vi "ACT_Loop.vi"() -> ()   [LabVIEW 2023, in "Swerve AM_ACT.lvlib"]
uses:
  Swerve AM_ACT.lvlib
  Cluster_CMD_ACT_Data.ctl
  ENUM_CMD_Mode Select.ctl
  Shared Code/TypeDefs/Cluster_CMD_Direction Data.ctl
  Shared Code/TypeDefs/Cluster_Module Velocity-Direction-Rotations.ctl
  Shared Code/TypeDefs/Level_Velocity plus-minus 1.ctl
  Shared Code/TypeDefs/Dial_Compase heading unit circle CCW positive.ctl
  Shared Code/TypeDefs/Cluster_X-Y.ctl
  Cluster_HW Output Values.ctl
  Shared Code/TypeDefs/Cluster_Swerve 4 Steer and Velocity.ctl
  Cluster_System Output Data.ctl
  Cluster_Config System Values.ctl
  Shared Code/TypeDefs/Cluster_SW PID Config.ctl
  Shared Code/TypeDefs/Cluster_PID Gains.ctl
  Shared Code/TypeDefs/Cluster_High-Low.ctl
  Type Defs/Cluster_Length and Width.ctl
  Shared Code/TypeDefs/Cluster_Config_SwerveParam Drive.ctl
  Shared Code/TypeDefs/Cluster_Config_SwerveParam Steer.ctl
  Cluster_Config Specific HW Values.ctl
  Cluster_Config Specific Data.ctl
  Shared Code/TypeDefs/ENUM_Module Position.ctl
  Cluster_Config Steer HW Values.ctl
  Shared Code/TypeDefs/Cluster_Config SRX Motor Output.ctl
  <vilib>/Rock Robotics/WPI/ThirdParty/Phoenix-LabVIEW/Motor Controller/Controls/CTRE_Phoenix_MotorControl_NeutralMode.ctl
  Shared Code/TypeDefs/Cluster_FWD  REV Values.ctl
  Shared Code/TypeDefs/Cluster_SRX SLOT PID Config.ctl
  Shared Code/TypeDefs/Cluster_SRX Motion Magic Parameters.ctl
  Cluster_Config Drive HW Values.ctl
  Shared Code/TypeDefs/Cluster_Spark MAX SLOT PID Config.ctl
  Shared Code/TypeDefs/Cluster_SparkMax Smart Motion Parameters.ctl
  ENUM_ACT_State.ctl
  <vilib>/Rock Robotics/WPI/ThirdParty/Phoenix-LabVIEW/Motor Controller/Controls/CTRE_Phoenix_MotorControl_ControlMode.ctl
  <vilib>/Rock Robotics/WPI/MotorControl/WPI_MotorControlDeviceRef.ctl
  <vilib>/Rock Robotics/WPI/MotorControl/WPI_MotorControlType.ctl
  <vilib>/Rock Robotics/SystemInterfaces/DIO/FPGA_DIOPWMChannel.ctl
  <vilib>/Rock Robotics/WPI/PWM/WPI_PWMDeadband.ctl
  <vilib>/Rock Robotics/SystemInterfaces/DIO/FPGA_DIOChannel.ctl
  ENUM_ACT_Action.ctl
  4f1f8321-3dc8-4b28-8619-20673fc77ec2.vi
  cbff3d61-3b62-444e-9844-795ae03579cd.vi
  089052c0-d540-4a78-a5cc-aeb70dbb496b.vi
  6201c2b1-dcd8-4430-86f1-9b4ee56c7753.vi
  b5508d6c-c1cc-4273-80c5-2077d34e1483.vi
  5f725c2a-0ce1-4524-8967-e83b15fdce90.vi
  bd5da564-2e8e-4505-86fc-30918feadaa2.vi
  8beda75f-c59a-4462-acc7-7c37ceab3777.vi
  47a9b741-f4a3-48b6-ae85-4ba2e502368e.vi
  e2e8a241-7810-4d95-85fd-17f3a55957a8.vi
  80d407e5-f582-430c-986f-ecd413765478.vi
  573e44c0-11f4-4bd9-ad56-904ec25dba75.vi
  e7494af9-f670-4352-9dfa-ae6ce50709ea.vi
  <vilib>/Utility/error.llb/Trim Whitespace.vi
  5f725c2a-0ce1-4524-8967-e83b15fdce90.vi/958b2683-dd4b-41b7-8ed1-41c95f63cef0.vi
  5f725c2a-0ce1-4524-8967-e83b15fdce90.vi/95f5fa9b-6175-4b34-88ee-cece92c38279.vi
  bd5da564-2e8e-4505-86fc-30918feadaa2.vi/958b2683-dd4b-41b7-8ed1-41c95f63cef0.vi
  bd5da564-2e8e-4505-86fc-30918feadaa2.vi/95f5fa9b-6175-4b34-88ee-cece92c38279.vi
  8beda75f-c59a-4462-acc7-7c37ceab3777.vi/958b2683-dd4b-41b7-8ed1-41c95f63cef0.vi
  8beda75f-c59a-4462-acc7-7c37ceab3777.vi/95f5fa9b-6175-4b34-88ee-cece92c38279.vi
  47a9b741-f4a3-48b6-ae85-4ba2e502368e.vi/958b2683-dd4b-41b7-8ed1-41c95f63cef0.vi
  47a9b741-f4a3-48b6-ae85-4ba2e502368e.vi/95f5fa9b-6175-4b34-88ee-cece92c38279.vi
  e2e8a241-7810-4d95-85fd-17f3a55957a8.vi/958b2683-dd4b-41b7-8ed1-41c95f63cef0.vi
  e2e8a241-7810-4d95-85fd-17f3a55957a8.vi/95f5fa9b-6175-4b34-88ee-cece92c38279.vi
  80d407e5-f582-430c-986f-ecd413765478.vi/958b2683-dd4b-41b7-8ed1-41c95f63cef0.vi
  80d407e5-f582-430c-986f-ecd413765478.vi/95f5fa9b-6175-4b34-88ee-cece92c38279.vi
  573e44c0-11f4-4bd9-ad56-904ec25dba75.vi/958b2683-dd4b-41b7-8ed1-41c95f63cef0.vi
  573e44c0-11f4-4bd9-ad56-904ec25dba75.vi/95f5fa9b-6175-4b34-88ee-cece92c38279.vi
  e7494af9-f670-4352-9dfa-ae6ce50709ea.vi/958b2683-dd4b-41b7-8ed1-41c95f63cef0.vi
  e7494af9-f670-4352-9dfa-ae6ce50709ea.vi/95f5fa9b-6175-4b34-88ee-cece92c38279.vi
  <vilib>/Utility/error.llb/Trim Whitespace One-Sided.vi
  5f725c2a-0ce1-4524-8967-e83b15fdce90.vi/95f5fa9b-6175-4b34-88ee-cece92c38279.vi/1c6bd52c-bbca-4d4a-a290-93ea2703fded.vi
  5f725c2a-0ce1-4524-8967-e83b15fdce90.vi/95f5fa9b-6175-4b34-88ee-cece92c38279.vi/47c2b0d5-b5fa-444e-9535-611565d375db.vi
  bd5da564-2e8e-4505-86fc-30918feadaa2.vi/95f5fa9b-6175-4b34-88ee-cece92c38279.vi/1c6bd52c-bbca-4d4a-a290-93ea2703fded.vi
  bd5da564-2e8e-4505-86fc-30918feadaa2.vi/95f5fa9b-6175-4b34-88ee-cece92c38279.vi/47c2b0d5-b5fa-444e-9535-611565d375db.vi
  8beda75f-c59a-4462-acc7-7c37ceab3777.vi/95f5fa9b-6175-4b34-88ee-cece92c38279.vi/1c6bd52c-bbca-4d4a-a290-93ea2703fded.vi
  8beda75f-c59a-4462-acc7-7c37ceab3777.vi/95f5fa9b-6175-4b34-88ee-cece92c38279.vi/47c2b0d5-b5fa-444e-9535-611565d375db.vi
  47a9b741-f4a3-48b6-ae85-4ba2e502368e.vi/95f5fa9b-6175-4b34-88ee-cece92c38279.vi/1c6bd52c-bbca-4d4a-a290-93ea2703fded.vi
  47a9b741-f4a3-48b6-ae85-4ba2e502368e.vi/95f5fa9b-6175-4b34-88ee-cece92c38279.vi/47c2b0d5-b5fa-444e-9535-611565d375db.vi
  e2e8a241-7810-4d95-85fd-17f3a55957a8.vi/95f5fa9b-6175-4b34-88ee-cece92c38279.vi/1c6bd52c-bbca-4d4a-a290-93ea2703fded.vi
  e2e8a241-7810-4d95-85fd-17f3a55957a8.vi/95f5fa9b-6175-4b34-88ee-cece92c38279.vi/47c2b0d5-b5fa-444e-9535-611565d375db.vi
  80d407e5-f582-430c-986f-ecd413765478.vi/95f5fa9b-6175-4b34-88ee-cece92c38279.vi/1c6bd52c-bbca-4d4a-a290-93ea2703fded.vi
  80d407e5-f582-430c-986f-ecd413765478.vi/95f5fa9b-6175-4b34-88ee-cece92c38279.vi/47c2b0d5-b5fa-444e-9535-611565d375db.vi
  573e44c0-11f4-4bd9-ad56-904ec25dba75.vi/95f5fa9b-6175-4b34-88ee-cece92c38279.vi/1c6bd52c-bbca-4d4a-a290-93ea2703fded.vi
  573e44c0-11f4-4bd9-ad56-904ec25dba75.vi/95f5fa9b-6175-4b34-88ee-cece92c38279.vi/47c2b0d5-b5fa-444e-9535-611565d375db.vi
  e7494af9-f670-4352-9dfa-ae6ce50709ea.vi/95f5fa9b-6175-4b34-88ee-cece92c38279.vi/1c6bd52c-bbca-4d4a-a290-93ea2703fded.vi
  e7494af9-f670-4352-9dfa-ae6ce50709ea.vi/95f5fa9b-6175-4b34-88ee-cece92c38279.vi/47c2b0d5-b5fa-444e-9535-611565d375db.vi
  RoboRIO Utilities/Global_STOP.vi
  Global_CMD_ACT_Data In.vi
  PigeonIMU/Global_SEN_Data Out.vi
  Global_ACT_Data Out.vi
  <vilib>/Utility/Data Type/Get Type Information.vi
  Shared Code/Utility/RWA/RWA/File/RWA_PC FIle Read String.vi
  Shared Code/Utility/RWA/RWA/Read Write Anything/RWA_File String.vi
  Shared Code/Utility/RWA/RWA/File/RWA_PC File Write String.vi
  <vilib>/Comparison/Equal/Equal Functor/Equal Functor.lvclass
  PigeonIMU/PigeonIMU_SEN_ts.lvlib
panel:
  in  "Set Steer Start Values":bool
  in  "Config Drive":T1={"Drive HW Ver"=0, "SparkMax Output"={"Idle Mode"=enum."Coast", "Ramp Rate (S)"=1.0}, "Slot 0 CL"={"Gains"={"P"=0.1, "I"=0.0, "D"=0.0, "F"=0.0}, "I Zone"=0.0, "Peak Out -1 0 1"={"High"=0.0, "Low"=0.0}, "Max I Accu"=0.0}, "Slot 0 SM"={"Max Velocity"=0.0, "Max Acceleration"=0.0, "Allowed CL Error"=0.0, "Min Velocity Output"=0.0}} {"Slot 0 CL"."Gains"."F" format="%#.8f"; "Slot 0 CL"."Gains"."D" format="%#.8f"; "Slot 0 CL"."Gains"."I" format="%#.8f"; "Slot 0 CL"."Gains"."P" format="%#.8f"; "Slot 0 CL"."Peak Out -1 0 1"."Low" format="%#.8f"; "Slot 0 CL"."Peak Out -1 0 1"."High" format="%#.8f"}
  in  "Config Steer":T6={"Steer HW Ver"=0, "SRX Output"={"Neutral"=enum."Override to Coast", "Max"={"FWD"=1.0, "REV"=-1.0}, "Min"={"FWD"=0.0, "REV"=0.0}, "OL Ramp Rate (S)"=0.0, "Dead Band"=0.0, "CL Ramp Rate (S)"=0.0}, "Slot 0 CL"={"Gains"={"P"=1.0, "I"=0.01, "D"=0.0, "F"=0.0}, "Error Allowed"=0.0, "I Zone"=10000.0, "Peak Out 0-1"=1.0, "Max I Accu"=-1000.0}, "Slot 0 MM"={"Cruise Velocity"=5000, "Acceleration"=5000}} {"Slot 0 CL"."Gains"."F" format="%#.8f"; "Slot 0 CL"."Gains"."D" format="%#.8f"; "Slot 0 CL"."Gains"."I" format="%#.8f"; "Slot 0 CL"."Gains"."P" format="%#.8f"; "SRX Output"."Min"."REV" format="%.2f"; "SRX Output"."Min"."FWD" format="%.2f"; "SRX Output"."Max"."REV" format="%.2f"; "SRX Output"."Max"."FWD" format="%.2f"}
  in  "Config Specific":T12={"Specific HW Ver"=0, "Specific Data"=[{"Motor Pos"=enum."Left-Front", "CAN Bus"="", "Drive ID"=0, "Drive Invert"=FALSE, "Steer ID"=0, "Steer Invert"=FALSE, "Encoder Start Value"=0.0}, {"Motor Pos"=enum."Right-Front", "CAN Bus"="", "Drive ID"=0, "Drive Invert"=FALSE, "Steer ID"=0, "Steer Invert"=FALSE, "Encoder Start Value"=0.0}, {"Motor Pos"=enum."Right-Back", "CAN Bus"="", "Drive ID"=0, "Drive Invert"=FALSE, "Steer ID"=0, "Steer Invert"=FALSE, "Encoder Start Value"=0.0}, {"Motor Pos"=enum."Left-Back", "CAN Bus"="", "Drive ID"=0, "Drive Invert"=FALSE, "Steer ID"=0, "Steer Invert"=FALSE, "Encoder Start Value"=0.0}]}
  in  "CMD Override":enum32{"None", "Mode 2", "Mode 1", "STOP"}(tab)
  in  "Mode 2 Data":dbl(slide) scale=-0.2..0.2
  in  "Mode 1 Data":i32
  in  "GO":bool
  out "Current Time":timestamp
  in  "Config System":T15={"System Ver"=0, "Auto Angle PID"={"Gains"={"P"=0.1, "I"=0.0, "D"=0.0, "F"=0.0}, "Error Allowed"={"High"=0.0, "Low"=0.0}, "I Zone"={"High"=0.0, "Low"=0.0}, "Peak Out 0-1"={"High"=0.0, "Low"=0.0}, "Max I Accu"={"High"=0.0, "Low"=0.0}}, "Frame"={"Length"=33.0, "Width"=18.0}, "DriveTrain"={"CPR"=14.0, "RevMotor/Wheel"=6.67, "Wheel Diameter (in)"=4.0}, "Speed Full Scale"=5000.0, "Steer Data"={"CPR"=1024.0}} {"Auto Angle PID"."Max I Accu"."Low" format="%#.8f"; "Auto Angle PID"."Max I Accu"."High" format="%#.8f"; "Auto Angle PID"."Gains"."F" format="%#.8f"; "Auto Angle PID"."Gains"."D" format="%#.8f"; "Auto Angle PID"."Gains"."I" format="%#.8f"; "Auto Angle PID"."Gains"."P" format="%#.8f"; "Auto Angle PID"."Error Allowed"."Low" format="%#.8f"; "Auto Angle PID"."Error Allowed"."High" format="%#.8f"; "Auto Angle PID"."I Zone"."Low" format="%#.8f"; "Auto Angle PID"."I Zone"."High" format="%#.8f"; "Auto Angle PID"."Peak Out 0-1"."Low" format="%#.8f"; "Auto Angle PID"."Peak Out 0-1"."High" format="%#.8f"}
  out "System Config":T20
  out "Sensor Read time":dbl format="%.3g"
  out "HW Output":T21 {"Swerve Read"."Back Right"."Angle" scale format="%.3f"; "Swerve Read"."Back Right"."Velocity" scale=-1.0..1.0 scale format="%.1f"; "Swerve Read"."Back Left"."Angle" scale format="%.3f"; "Swerve Read"."Back Left"."Velocity" scale=-1.0..1.0 scale format="%.1f"; "Swerve Read"."Front Left"."Angle" scale format="%.3f"; "Swerve Read"."Front Left"."Velocity" scale=-1.0..1.0 scale format="%.1f"; "Swerve Read"."Front Right"."Angle" scale format="%.3f"; "Swerve Read"."Front Right"."Velocity" scale=-1.0..1.0 scale format="%.1f"; "Pigeon Heading" scale format="%.3f"}
  in  "Read Saved Config":bool
  in  "Update Config":bool
  out "CMD":T26 {"Target Auto Angle" scale format="%.3f"; "Direction"."Rotate(Yaw) CCW 1 CW -1" scale=1.0..-1.0; "Direction"."Traverse"."Angle" scale format="%.3f"; "Direction"."Traverse"."Velocity" scale=-1.0..1.0 scale format="%.1f"}
  out "Cycle Time (S)":dbl format="%.3g"
  # "STOP"
  # "\"Front\" of Robot"
  # "Right Hand Rule"
  # "X"
  # "+CCW"
  # "Y"
  # "(0,0)"
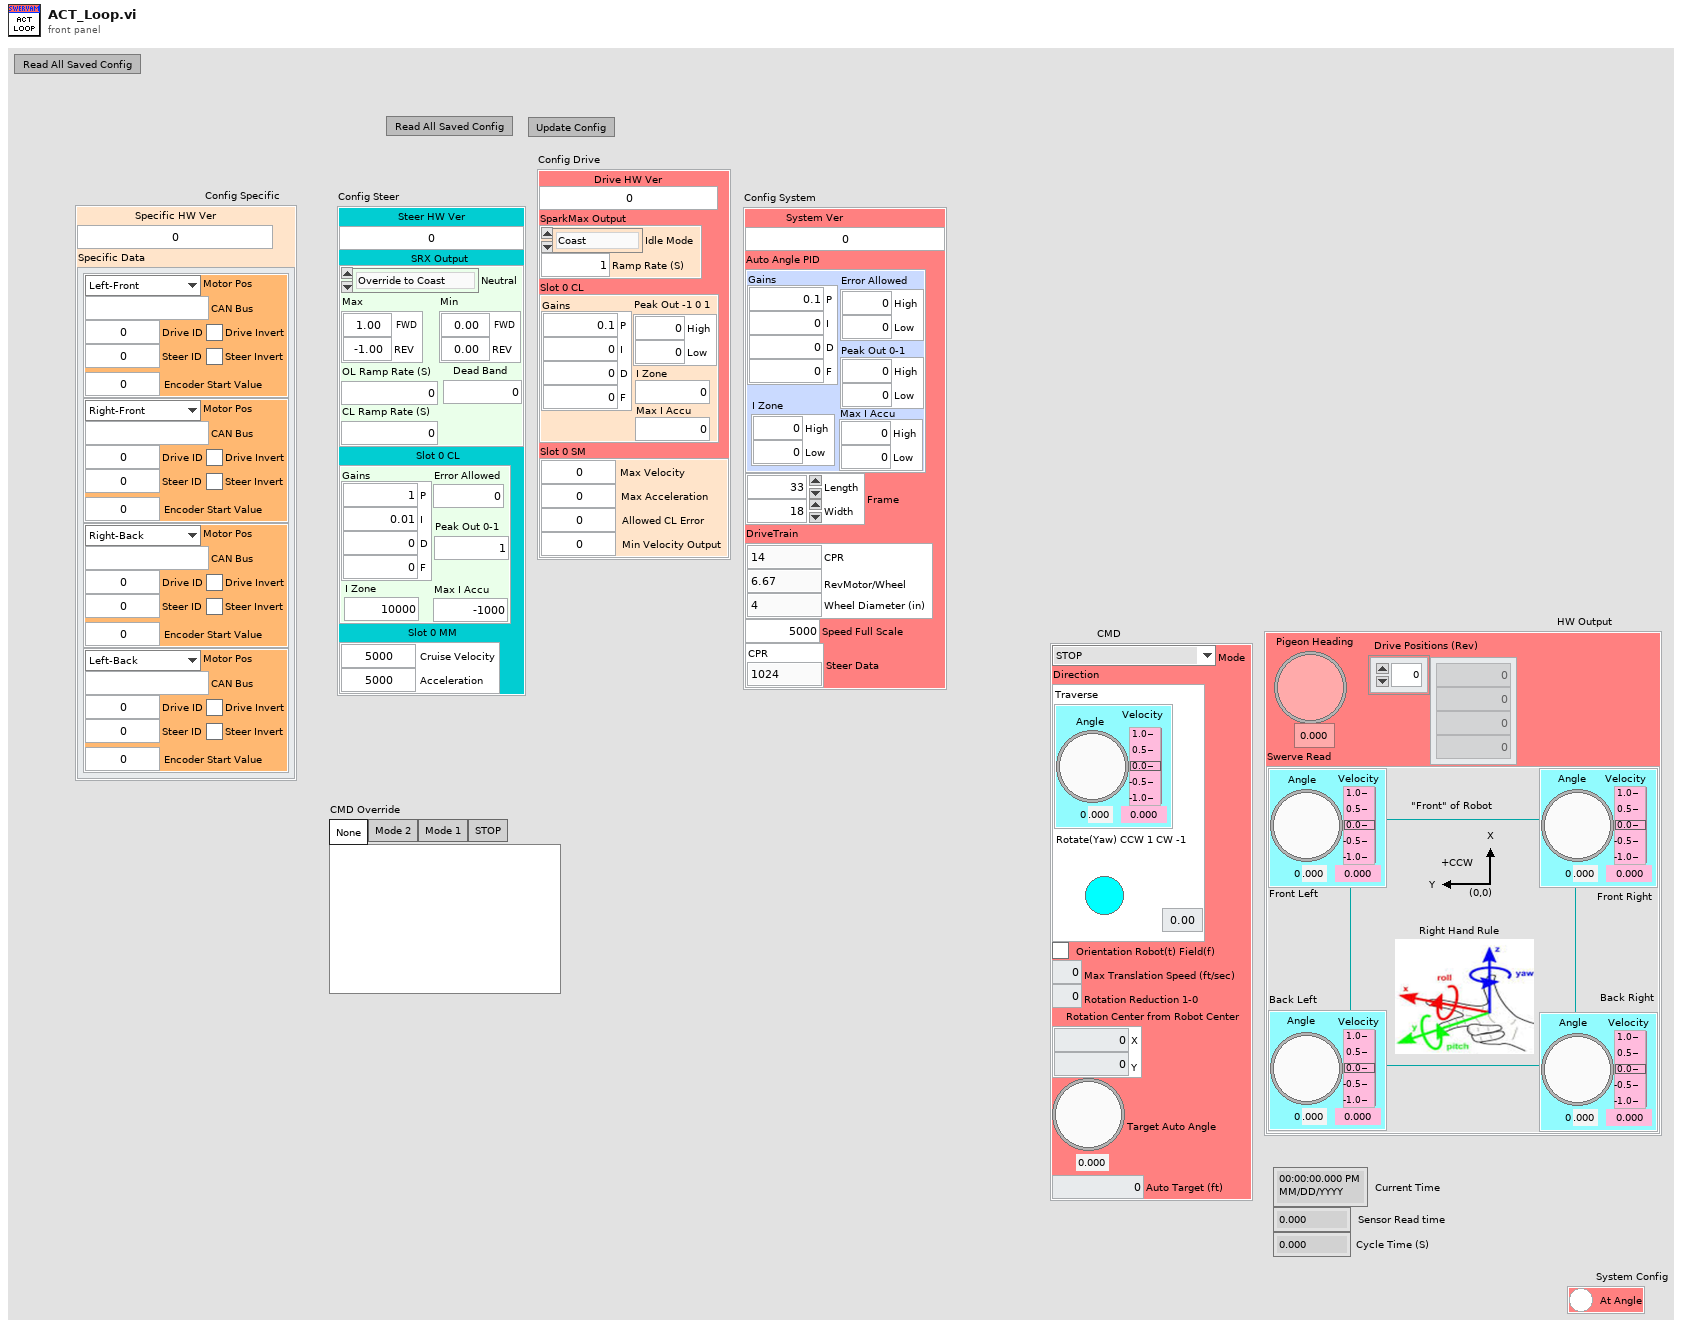
[diagram p1: front panel]
types:
  T1 = typedef "Swerve AM_ACT.lvlib/Cluster_Config Drive HW Values.ctl" = cluster{"Drive HW Ver":u64, "SparkMax Output":cluster{"Idle Mode":enum16{"Coast", "Brake"}, "Ramp Rate (S)":dbl}, "Slot 0 CL":T2, "Slot 0 SM":T5}
  T2 = typedef "Cluster_Spark MAX SLOT PID Config.ctl" = cluster{"Gains":T3, "I Zone":dbl, "Peak Out -1 0 1":T4, "Max I Accu":dbl}
  T3 = typedef "Cluster_PID Gains.ctl" = cluster{"P":dbl, "I":dbl, "D":dbl, "F":dbl}
  T4 = typedef "Cluster_High-Low.ctl" = cluster{"High":dbl, "Low":dbl}
  T5 = typedef "Cluster_SparkMax Smart Motion Parameters.ctl" = cluster{"Max Velocity":dbl, "Max Acceleration":dbl, "Allowed CL Error":dbl, "Min Velocity Output":dbl}
  T6 = typedef "Swerve AM_ACT.lvlib/Cluster_Config Steer HW Values.ctl" = cluster{"Steer HW Ver":u64, "SRX Output":T7, "Slot 0 CL":T10, "Slot 0 MM":T11}
  T7 = typedef "Cluster_Config SRX Motor Output.ctl" = cluster{"Neutral":T8, "Max":T9, "Min":T9, "OL Ramp Rate (S)":dbl, "Dead Band":dbl, "CL Ramp Rate (S)":dbl}
  T8 = typedef "CTRE_Phoenix_MotorControl_NeutralMode.ctl" = enum8{"EEPROMSetting", "Override to Coast", "Override to Brake"}
  T9 = typedef "Cluster_FWD  REV Values.ctl" = cluster{"FWD":dbl, "REV":dbl}
  T10 = typedef "Cluster_SRX SLOT PID Config.ctl" = cluster{"Gains":T3, "Error Allowed":dbl, "I Zone":dbl, "Peak Out 0-1":dbl, "Max I Accu":dbl}
  T11 = typedef "Cluster_SRX Motion Magic Parameters.ctl" = cluster{"Cruise Velocity":i32, "Acceleration":i32}
  T12 = typedef "Swerve AM_ACT.lvlib/Cluster_Config Specific HW Values.ctl" = cluster{"Specific HW Ver":u64, "Specific Data":T13[]}
  T13 = typedef "Swerve AM_ACT.lvlib/Cluster_Config Specific Data.ctl" = cluster{"Motor Pos":T14, "CAN Bus":string, "Drive ID":u8, "Drive Invert":bool, "Steer ID":u8, "Steer Invert":bool, "Encoder Start Value":dbl}
  T14 = typedef "ENUM_Module Position.ctl" = enum16{"Left-Front", "Right-Front", "Left-Back", "Right-Back"}
  T15 = typedef "Swerve AM_ACT.lvlib/Cluster_Config System Values.ctl" = cluster{"System Ver":u64, "Auto Angle PID":T16, "Frame":T17, "DriveTrain":T18, "Speed Full Scale":dbl, "Steer Data":T19}
  T16 = typedef "Cluster_SW PID Config.ctl" = cluster{"Gains":T3, "Error Allowed":T4, "I Zone":T4, "Peak Out 0-1":T4, "Max I Accu":T4}
  T17 = typedef "Cluster_Length and Width.ctl" = cluster{"Length":dbl, "Width":dbl}
  T18 = typedef "Cluster_Config_SwerveParam Drive.ctl" = cluster{"CPR":dbl, "RevMotor/Wheel":dbl, "Wheel Diameter (in)":dbl}
  T19 = typedef "Cluster_Config_SwerveParam Steer.ctl" = cluster{"CPR":dbl}
  T20 = typedef "Swerve AM_ACT.lvlib/Cluster_System Output Data.ctl" = cluster{"At Angle":bool}
  T21 = typedef "Swerve AM_ACT.lvlib/Cluster_HW Output Values.ctl" = cluster{"Pigeon Heading":T22, "Swerve Read":T23, "Drive Positions (Rev)":dbl[]}
  T22 = typedef "Dial_Compase heading unit circle CCW positive.ctl" = dbl
  T23 = typedef "Cluster_Swerve 4 Steer and Velocity.ctl" = cluster{"Front Right":T24, "Front Left":T24, "Back Left":T24, "Back Right":T24}
  T24 = typedef "Cluster_Module Velocity-Direction-Rotations.ctl" = cluster{"Velocity":T25, "Angle":T22, "Rotations Count":dbl}
  T25 = typedef "Level_Velocity plus-minus 1.ctl" = dbl
  T26 = typedef "Swerve AM_ACT.lvlib/Cluster_CMD_ACT_Data.ctl" = cluster{"Mode":T27, "Direction":T28, "Orientation Robot(t) Field(f)":bool, "Max Translation Speed (ft/sec)":dbl, "Rotation Reduction 1-0":dbl, "Rotation Center from Robot Center":T29, "Target Auto Angle":T22, "Auto Target (ft)":dbl}
  T27 = typedef "Swerve AM_ACT.lvlib/ENUM_CMD_Mode Select.ctl" = enum16{"STOP", "Move", "Turret Manual", "Trans Manual Angle Auto", "Turret Auto Angle"}
  T28 = typedef "Cluster_CMD_Direction Data.ctl" = cluster{"Traverse":T24, "Rotate(Yaw) CCW 1 CW -1":dbl}
  T29 = typedef "Cluster_X-Y.ctl" = cluster{"X":dbl, "Y":dbl}
  T30 = typedef "WPI_MotorControlDeviceRef.ctl" = cluster{"DeviceStatus":errorcluster, "Type":T31, "PWM":cluster{"PWM Channel":T32, "DeadBand":T33}, "CAN":cluster{"Device Number":u8, "SetOutput VI Ref":variant, "GetOutput VI Ref":variant, "Enable VI Ref":variant, "Disable VI Ref":variant, "Data":variant}, "Invert":bool, "DIO PWM":cluster{"PWM \"Enable\" Channel":T32, "DIOChannel":T34, "PWM Rate":dbl}}
  T31 = typedef "WPI_MotorControlType.ctl" = enum16{"PWM", "CAN", "DIO PWM"}
  T32 = typedef "FPGA_DIOPWMChannel.ctl" = enum8{"PWM 0", "PWM 1", "PWM 2", "PWM 3", "PWM 4", "PWM 5", "PWM 6", "PWM 7", "PWM 8", "PWM 9", "PWM MXP 0", "PWM MXP 1", "PWM MXP 2", "PWM MXP 3", "PWM MXP 4", "PWM MXP 5", "PWM MXP 6", "PWM MXP 7", "PWM MXP 8", "PWM MXP 9", "Invalid"}
  T33 = typedef "WPI_PWMDeadband.ctl" = cluster{"Name":string, "maxPositivePwm":i32, "minPositivePwm":i32, "centerPwm":i32, "maxNegativePwm":i32, "minNegativePwm":i32, "angularRange":u16}
  T34 = typedef "FPGA_DIOChannel.ctl" = enum8{"DIO 0", "DIO 1", "DIO 2", "DIO 3", "DIO 4", "DIO 5", "DIO 6", "DIO 7", "DIO 8", "DIO 9", "DIO MXP 0", "DIO MXP 1", "DIO MXP 2", "DIO MXP 3", "DIO MXP 4", "DIO MXP 5", "DIO MXP 6", "DIO MXP 7", "DIO MXP 8", "DIO MXP 9", "DIO MXP 10", "DIO MXP 11", "DIO MXP 12", "DIO MXP 13", "DIO MXP 14", "DIO MXP 15", "SPI Port CS1", "SPI Port CS2", "SPI Port CS3", "SPI Port MISO", "SPI Port MOSI", "Invalid"}
  T35 = typedef "CTRE_Phoenix_MotorControl_ControlMode.ctl" = u16
  T36 = typedef "Swerve AM_ACT.lvlib/ENUM_ACT_State.ctl" = enum16{"Startup", "Configuring", "Stopping", "Moving Mode 1", "Moving Mode 2", "Shutdown", "Initializing HW"}
  T37 = cluster{"Motor List":T14[], "Team Folder":path, "FX Ref":T30, "Steer Refs":T30[], "Drive Refs":T30[], "State":T36, "Previous State":T36, "Current Time":timestamp, "Previous Time":timestamp, "Start Time":timestamp, "Target Time (ms)":u32, "Cycle Time(S)":dbl, "Update Display":bool, "ACT Input":T26, "Config System":T15, "Max # Of Config Tries":i32, "HW Out":T21, "System Output":T20, "CAN Timeout":u32, "FX Mode":T35, "FX Set Value":dbl, "Config Specific":T12, "Swerve Set":T23, "New Cmd":bool, "Config Steer":T6, "Config Drive":T1, "HW OPEN":bool, "Steer Change":bool, "Drive Change":bool, "Specific Change":bool, "System Change":bool}
  T38 = typedef "Swerve AM_ACT.lvlib/ENUM_ACT_Action.ctl" = enum16{"No Action", "Reset Time", "Reset All", "Open HW References", "Control FX Stop", "Control FX Mode 1", "Control FX Mode 2", "Set Robot Start Position", "Config HW Steer Set", "Config HW Steer Get", "Config HW Steer Save", "Config HW Steer Read", "Config HW Drive Set", "Config HW Drive Get", "Config HW Drive Save", "Config HW Drive Read", "Config HW Specific Set", "Config HW Specific Get", "Config HW Specific Save", "Config HW Specific Read", "Config System Save", "Config System Read", "Config From FP", "Start HW Steer Set", "Default HW Steer Set", "Defalut HW Drive Set"}
  T39 = cluster{"[0]":T24, "[1]":T24, "[2]":T24, "[3]":T24}
  T40 = typedef "Cluster_Unity Yaw-Pitch-Roll.ctl" = cluster{"Yaw":T22, "Pitch":T22, "Roll":T22}
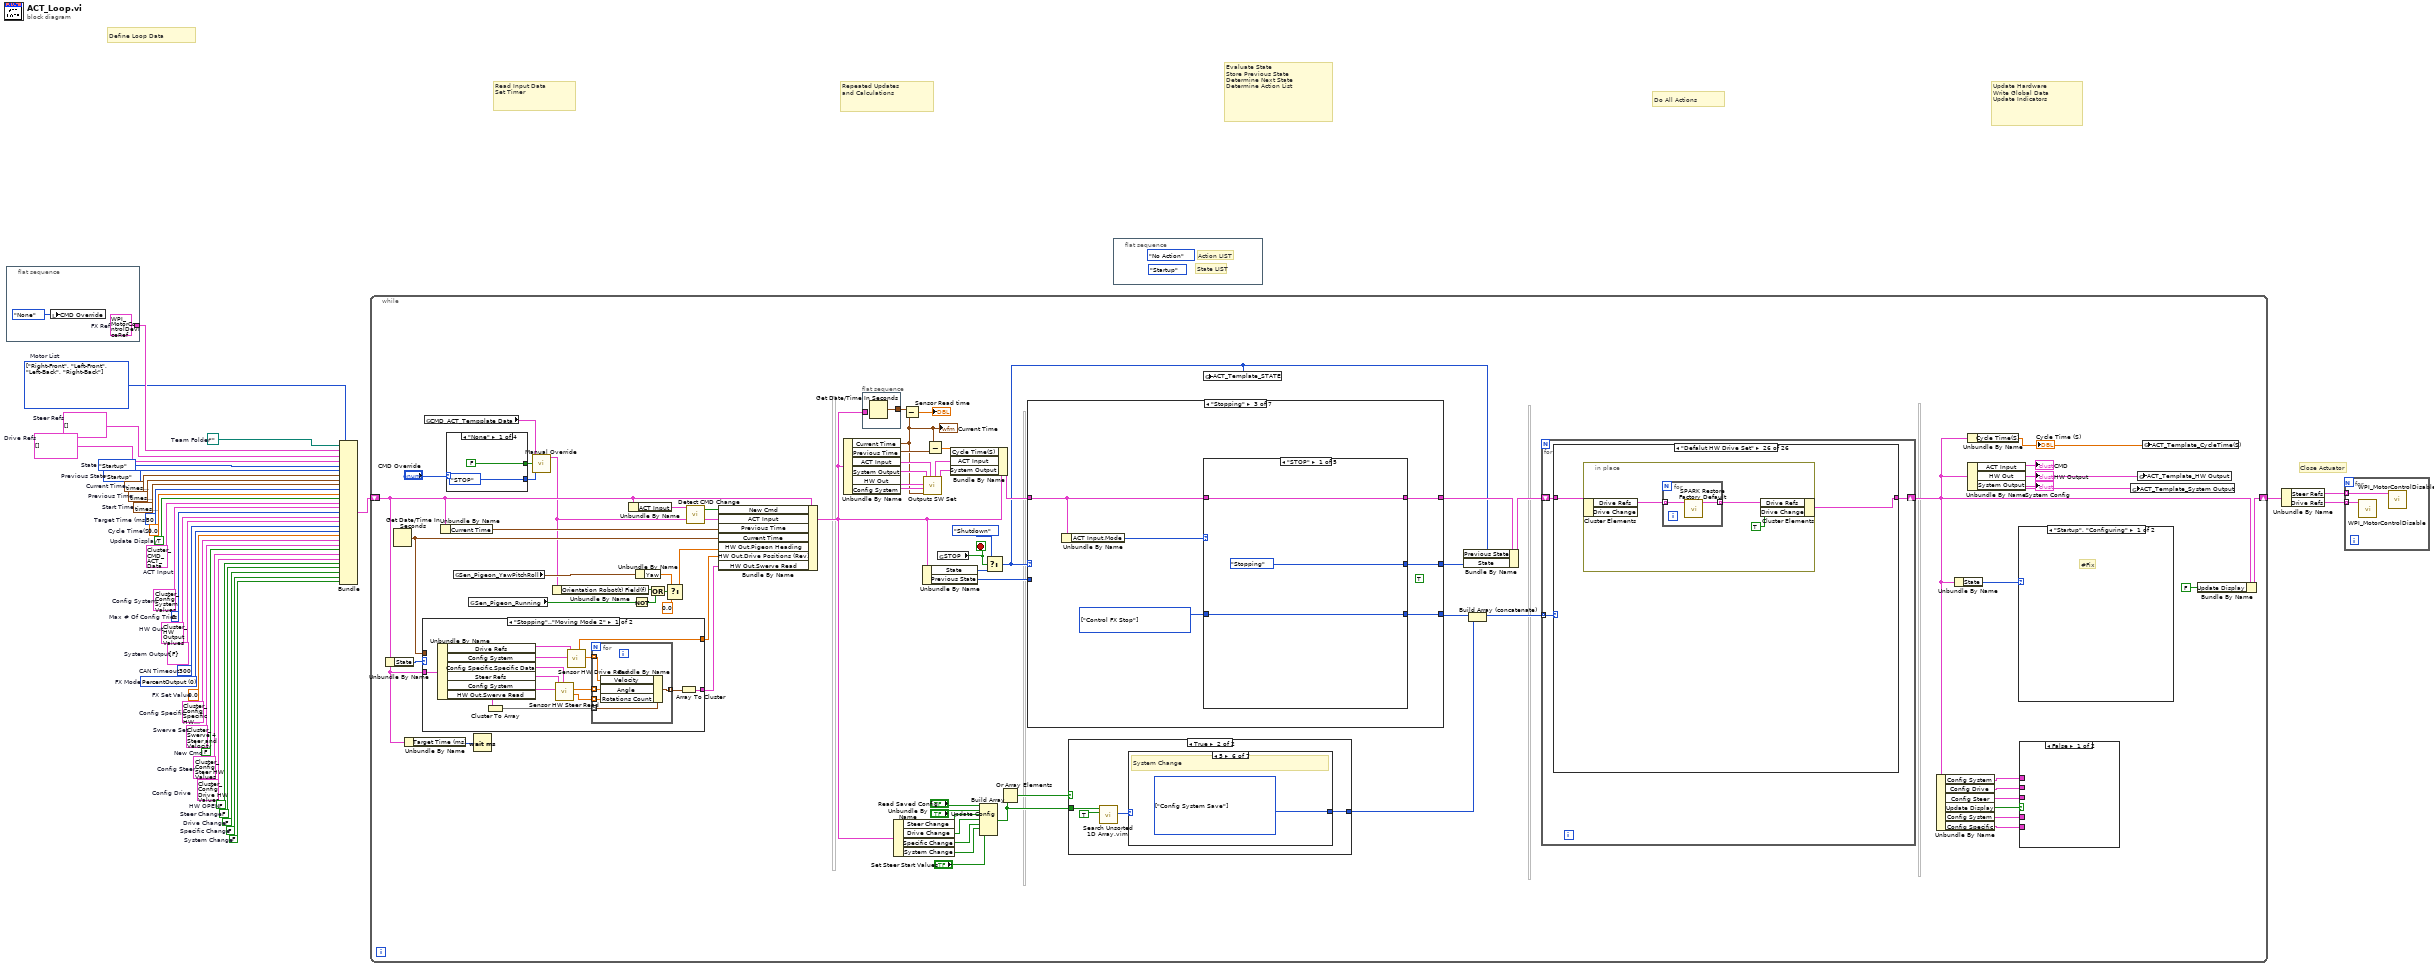
[diagram p0: block diagram]
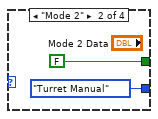
[diagram p2: hidden frame]
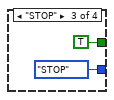
[diagram p3: hidden frame]
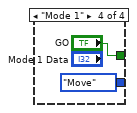
[diagram p4: hidden frame]
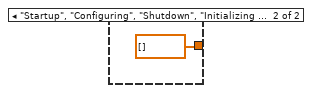
[diagram p5: hidden frame]
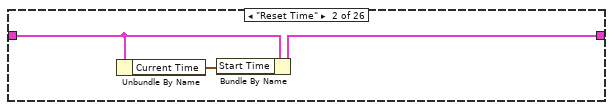
[diagram p7: hidden frame]
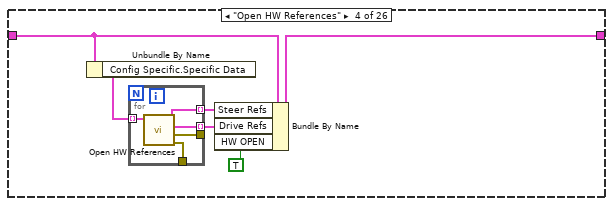
[diagram p9: hidden frame]
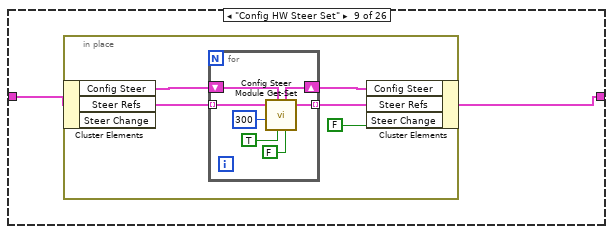
[diagram p14: hidden frame]
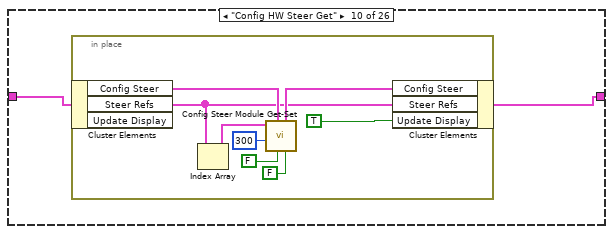
[diagram p15: hidden frame]
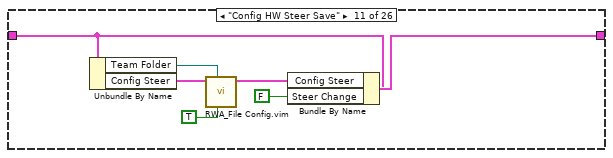
[diagram p16: hidden frame]
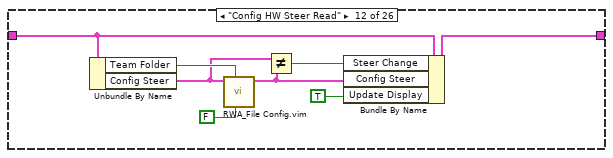
[diagram p17: hidden frame]
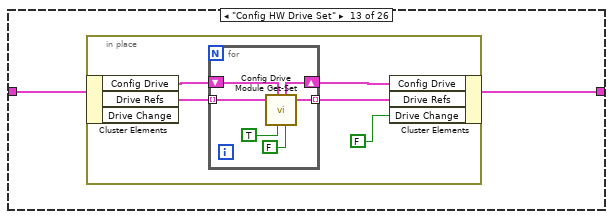
[diagram p18: hidden frame]
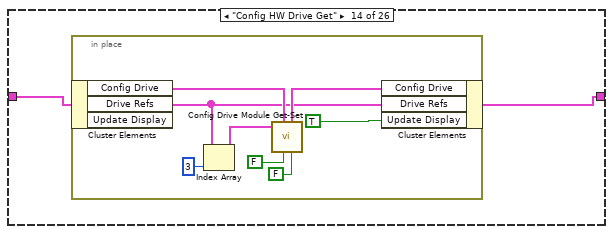
[diagram p19: hidden frame]
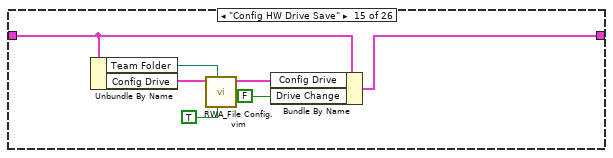
[diagram p20: hidden frame]
diagram:
  w1 = FALSE  # System Change
  w2 = FALSE  # Specific Change
  w3 = FALSE  # Drive Change
  w4 = FALSE  # Steer Change
  w5 = FALSE  # HW OPEN
  w7 = T6 {"Steer HW Ver"=0, "SRX Output"={"Neutral"=enum."Override to Coast", "Max"={"FWD"=1.0, "REV"=-1.0}, "Min"={"FWD"=0.0, "REV"=0.0}, "OL Ramp Rate (S)"=0.0, "Dead Band"=0.0, "CL Ramp Rate (S)"=0.0}, "Slot 0 CL"={"Gains"={"P"=1.0, "I"=0.01, "D"=0.0, "F"=0.0}, "Error Allowed"=0.0, "I Zone"=10000.0, "Peak Out 0-1"=1.0, "Max I Accu"=-1000.0}, "Slot 0 MM"={"Cruise Velocity"=5000, "Acceleration"=5000}}  # Config Steer
  w6 = T1 {"Drive HW Ver"=0, "SparkMax Output"={"Idle Mode"=enum."Coast", "Ramp Rate (S)"=1.0}, "Slot 0 CL"={"Gains"={"P"=0.1, "I"=0.0, "D"=0.0, "F"=0.0}, "I Zone"=0.0, "Peak Out -1 0 1"={"High"=0.0, "Low"=0.0}, "Max I Accu"=0.0}, "Slot 0 SM"={"Max Velocity"=0.0, "Max Acceleration"=0.0, "Allowed CL Error"=0.0, "Min Velocity Output"=0.0}}  # Config Drive
  w8 = FALSE  # New Cmd
  w9 = path ""  # Team Folder
  w11 = T23 {"Front Right"={"Velocity"=0.0, "Angle"=0.0, "Rotations Count"=0.0}, "Front Left"={"Velocity"=0.0, "Angle"=0.0, "Rotations Count"=0.0}, "Back Left"={"Velocity"=0.0, "Angle"=0.0, "Rotations Count"=0.0}, "Back Right"={"Velocity"=0.0, "Angle"=0.0, "Rotations Count"=0.0}}  # Swerve Set
  w12 = T14[] [enum."Right-Front", enum."Left-Front", enum."Left-Back", enum."Right-Back"] items=["Left-Front", "Right-Front", "Left-Back", "Right-Back"]  # Motor List
  w15 = T30[] []  # Steer Refs
  w14 = T30[] []  # Drive Refs
  w16 = T12 {"Specific HW Ver"=0, "Specific Data"=[{"Motor Pos"=enum."Left-Front", "CAN Bus"="", "Drive ID"=0, "Drive Invert"=FALSE, "Steer ID"=0, "Steer Invert"=FALSE, "Encoder Start Value"=0.0}, {"Motor Pos"=enum."Right-Front", "CAN Bus"="", "Drive ID"=0, "Drive Invert"=FALSE, "Steer ID"=0, "Steer Invert"=FALSE, "Encoder Start Value"=0.0}, {"Motor Pos"=enum."Right-Back", "CAN Bus"="", "Drive ID"=0, "Drive Invert"=FALSE, "Steer ID"=0, "Steer Invert"=FALSE, "Encoder Start Value"=0.0}, {"Motor Pos"=enum."Left-Back", "CAN Bus"="", "Drive ID"=0, "Drive Invert"=FALSE, "Steer ID"=0, "Steer Invert"=FALSE, "Encoder Start Value"=0.0}]}  # Config Specific
  w22 = T20 {"At Angle"=FALSE}  # System Output
  w24 = T15 {"System Ver"=0, "Auto Angle PID"={"Gains"={"P"=0.2, "I"=0.0, "D"=0.0, "F"=0.0}, "Error Allowed"={"High"=0.0, "Low"=0.0}, "I Zone"={"High"=0.0, "Low"=0.0}, "Peak Out 0-1"={"High"=0.0, "Low"=0.0}, "Max I Accu"={"High"=0.0, "Low"=0.0}}, "Frame"={"Length"=33.0, "Width"=18.0}, "DriveTrain"={"CPR"=14.0, "RevMotor/Wheel"=6.67, "Wheel Diameter (in)"=4.0}, "Speed Full Scale"=5000.0, "Steer Data"={"CPR"=1024.0}}  # Config System
  w23 = T21 {"Pigeon Heading"=0.0, "Swerve Read"={"Front Right"={"Velocity"=0.0, "Angle"=0.0, "Rotations Count"=0.0}, "Front Left"={"Velocity"=0.0, "Angle"=0.0, "Rotations Count"=0.0}, "Back Left"={"Velocity"=0.0, "Angle"=0.0, "Rotations Count"=0.0}, "Back Right"={"Velocity"=0.0, "Angle"=0.0, "Rotations Count"=0.0}}, "Drive Positions (Rev)"=[]}  # HW Out
  w19 = 0.0  # FX Set Value
  w20 = T35 0 items=["PercentOutput"=0, "Position"=1, "Velocity"=2, "Current"=3, "Follower"=5, "MotionProfile"=6, "MotionMagic"=7, "MotionProfileArc"=10, "Disabled"=15]  # FX Mode
  w18 = u32 300  # CAN Timeout
  w17 = 3  # Max # Of Config Tries
  w26 = TRUE  # Update Display
  w29 = 0.0  # Cycle Time(S)
  w30 = ENUM_ACT_State."Startup"  # Previous State
  w31 = timestamp(0 s since 1904-01-01)  # Previous Time
  w32 = u32 50  # Target Time (ms)
  w21 = T26 {"Mode"=enum."STOP", "Direction"={"Traverse"={"Velocity"=0.0, "Angle"=0.0, "Rotations Count"=0.0}, "Rotate(Yaw) CCW 1 CW -1"=0.0}, "Orientation Robot(t) Field(f)"=FALSE, "Max Translation Speed (ft/sec)"=0.0, "Rotation Reduction 1-0"=0.0, "Rotation Center from Robot Center"={"X"=0.0, "Y"=0.0}, "Target Auto Angle"=0.0, "Auto Target (ft)"=0.0}  # ACT Input
  w33 = timestamp(0 s since 1904-01-01)  # Start Time
  w34 = timestamp(0 s since 1904-01-01)  # Current Time
  w35 = ENUM_ACT_State."Startup"  # State
  # "Close Actuator"
  # "Define Loop Data"
  # "Repeated Updates\nand Calculations"
  # "Read Input Data\nSet Timer"
  # "Evaluate State\nStore Previous State\nDetermine Next State\nDetermine Action List"
  # "Do All Actions"
  # "Update Hardware\nWrite Global Data\nUpdate Indicators"
  n1 = flat-sequence {
    tunnel: [w37] -> w27
    frame #0 {
      w37 = T30 {"DeviceStatus"={"status"=FALSE, "code"=0, "source"=""}, "Type"=enum."PWM", "PWM"={"PWM Channel"=enum."PWM 1", "DeadBand"={"Name"="", "maxPositivePwm"=0, "minPositivePwm"=0, "centerPwm"=0, "maxNegativePwm"=0, "minNegativePwm"=0, "angularRange"=0}}, "CAN"={"Device Number"=0, "SetOutput VI Ref"=variant(enum8{"Percent VBus", "Current", "Speed", "Position", "Voltage"} enum."Percent VBus"), "GetOutput VI Ref"=variant(refnum<k1> refnum), "Enable VI Ref"=variant(dbl 12.0), "Disable VI Ref"=variant(enum8{"Percent VBus", "Speed", "Position", "Slave", "Unchanged / Invalid", "Voltage Compensation", "Current", "Motion Profile"} enum."Percent VBus"), "Data"=variant}, "Invert"=FALSE, "DIO PWM"={"PWM \"Enable\" Channel"=enum."Invalid", "DIOChannel"=enum."Invalid", "PWM Rate"=0.0}}  # FX Ref
      n2 = local write "CMD Override"(enum32{"None", "Mode 2", "Mode 1", "STOP"}."None" ("CMD Override")) -> ()
    }
  }
  n3 = Bundle("Motor List"=w12, "Team Folder"=w9, "FX Ref"=w27, "Steer Refs"=w15, "Drive Refs"=w14, "State"=w35, "Previous State"=w30, "Current Time"=w34, "Previous Time"=w31, "Start Time"=w33, "Target Time (ms)"=w32, "Cycle Time(S)"=w29, "Update Display"=w26, "ACT Input"=w21, "Config System"=w24, "Max # Of Config Tries"=w17, "HW Out"=w23, "System Output"=w22, "CAN Timeout"=w18, "FX Mode"=w20, "FX Set Value"=w19, "Config Specific"=w16, "Swerve Set"=w11, "New Cmd"=w8, "Config Steer"=w7, "Config Drive"=w6, "HW OPEN"=w5, "Steer Change"=w4, "Drive Change"=w3, "Specific Change"=w2, "System Change"=w1) -> (w10:T37)  [unwired: 1 in]
  n4 = while {
    shift-right: [w92] -> w28
    shift-left: w10 -> [w50]
    stop <- w103 stop-if-true
    n5 = Unbundle By Name(w50) -> ("State"=w84:T36)
    n6 = Get Date/Time In Seconds() -> (seconds since 1Jan1904=w80:timestamp)
    n7 = Unbundle By Name(w50) -> ("Target Time (ms)"=w100:u32)
    n8 = case shown="\"Stopping\"..\"Moving Mode 2\"" w84 {
      tunnel: w50 -> [w127 _]
      tunnel: w80 -> [_ _]
      tunnel: [w122 _] -> w51
      tunnel: [w117 dbl[] [] ("Drive Positions (Rev) Out")] -> w52
      frame "Stopping".."Moving Mode 2" {
        n9 = Unbundle By Name(w127) -> ("Drive Refs"=w128:T30[], "Config System"=w125:T15, "Config Specific.Specific Data"=w126:T13[], "Steer Refs"=w129:T30[], "Config System"=w116:T15, "HW Out.Swerve Read"=w124:T23)
        n10 = Cluster To Array(cluster=w124) -> (array=w123:T24[])
        n11 = call "Sensor HW Steer Read.vi"("HW Specific Config.Specific Data"=w126, "Steer"=w116, "Steer Ref"=w129) -> ("Offsets Out"=w118:dbl[], "Angles Out"=w119:dbl[])  [unwired: 5 in, 2 out]
        n12 = call "Sensor HW Drive Read.vi"("Config HW Drive Values"=w125, "Drive Ref"=w128) -> ("Drive Velocities (0-1) Out"=w120:dbl[], "Drive Positions (Rev) Out"=w117:dbl[])  [unwired: 6 in, 2 out]
        n13 = for {
          tunnel: w123 -> [w134] mode=indexing
          tunnel: [w133] -> w121 mode=indexing
          tunnel: w120 -> [w132] mode=indexing
          tunnel: w119 -> [w131] mode=indexing
          tunnel: w118 -> [w130] mode=indexing
          n14 = Bundle By Name(cluster=w134, "Velocity"=w132, "Angle"=w131, "Rotations Count"=w130) -> (w133:T24)
        }
        n15 = Array To Cluster(array=w121) -> (cluster=w122:T39)
      }
      frame "Startup", "Configuring", "Shutdown", "Initializing HW" {
      }
    }
    n16 = global read "Global_CMD_ACT_Data In.vi" "CMD_ACT_Tempplate Data"() -> (w57:T26)
    n17 = Unbundle By Name(w50) -> ("Current Time"=w99:timestamp)
    n18 = case shown="\"None\"" "CMD Override" {
      tunnel: [FALSE ("Enable") FALSE ("Enable") TRUE ("Positon GO") "GO"] -> w67
      tunnel: [ENUM_CMD_Mode_Select."STOP" ("Override") ENUM_CMD_Mode_Select."Turret Manual" ("Override") ENUM_CMD_Mode_Select."STOP" ("Override") ENUM_CMD_Mode_Select."Move" ("Override")] -> w66
      frame "None" {
      }
      frame "Mode 2" {
      }
      frame "STOP" {
      }
      frame "Mode 1" {
      }
    }
    n19 = global read "Global_SEN_Data Out.vi" "Sen_Pigeon_YawPitchRoll"() -> (w63:T40)
    n20 = global read "Global_SEN_Data Out.vi" "Sen_Pigeon_Running"() -> (w60:bool)
    n21 = Wait (ms)(milliseconds to wait=w100) -> ()  [unwired: 1 out]
    n22 = call "Manual Override.vi"("Override"=w66, "Enable"=w67, "Auto CMD"=w57) -> ("OverRide Command Out"=w48:T26)  [unwired: 8 in]
    n23 = Unbundle By Name(w48) -> ("Orientation Robot(t) Field(f)"=w64:bool)
    n24 = Unbundle By Name(w50) -> ("ACT Input"=w49:T26)
    n25 = Not(x=w60) -> (.not. x?=w59:bool)
    n26 = Unbundle By Name(w63) -> ("Yaw"=w58:T22)
    n27 = Or(x=w64, y=w59) -> (x .or. y?=w61:bool)
    n28 = Select(t=T22 0.0, s=w61, f=w58) -> (s? t:f=w56:T22)
    n29 = call "Detect CMD Change.vi"("CMD_ACT_SwerveDrive_Data"=w48, "Preious ACT Input"=w49) -> ("New Command"=w47:bool)  [unwired: 9 in]
    n30 = Bundle By Name(cluster=w50, "New Cmd"=w47, "ACT Input"=w48, "Previous Time"=w99, "Current Time"=w80, "HW Out.Pigeon Heading"=w56, "HW Out.Drive Positions (Rev)"=w52, "HW Out.Swerve Read"=w51) -> (w43:T37)
    n31 = Unbundle By Name(w43) -> ("Current Time"=w44:timestamp, "Previous Time"=w97:timestamp, "ACT Input"=w55:T26, "System Output"=w73:T20, "HW Out"=w71:T21, "Config System"=w70:T15)
    "Current Time" <- w44
    n32 = flat-sequence {
      tunnel: [w115] -> w82
      tunnel: w43 -> [_]
      frame #0 {
        n33 = Get Date/Time In Seconds() -> (seconds since 1Jan1904=w115:timestamp)
      }
    }
    n34 = Unbundle By Name(w43) -> ("Steer Change"=w42:bool, "Drive Change"=w41:bool, "Specific Change"=w40:bool, "System Change"=w39:bool)
    n35 = Subtract(x=w82, y=w44) -> (x-y=→"Sensor Read time":dbl)
    n36 = Unbundle By Name(w43) -> ("State"=w101:T36, "Previous State"=w98:T36)
    n37 = call "Outputs SW Set.vi"("Auto CMD"=w55, "Current Time"=w44, "System Config"=w70, "Sensor Values"=w71, "SW Output"=w73) -> ("SW Output Out"=w72:T20, "Auto CMD Out"=w54:T26)  [unwired: 5 in]
    n38 = Subtract(x=w44, y=w97) -> (x-y=w95:dbl)
    n39 = global read "Global_STOP.vi" "STOP"() -> (w103:bool)
    n40 = Bundle By Name(cluster=w43, "Cycle Time(S)"=w95, "ACT Input"=w54, "System Output"=w72) -> (w96:T37)
    n41 = Build Array("Read Saved Config", "Update Config", w42, w41, w40, w39, "Set Steer Start Values") -> (w76:bool[])
    n42 = Select(t=ENUM_ACT_State."Shutdown" ("State"), s=w103, f=w101) -> (s? t:f=w65:T36)
    n43 = Or Array Elements(Boolean array=w76) -> (logical OR=w77:bool)
    n44 = case shown="\"Stopping\"" w65 {
      selector: w65 -> [_ _ _ _ w432 w454 _]
      tunnel: w96 -> [w335 w349 w392 w413 w433 w455 w476]
      tunnel: [w336 w349 w391 w412 w434 w456 w476] -> w105
      tunnel: [ENUM_ACT_State."Configuring" ("State") w360 w390 w411 w436 w458 ENUM_ACT_State."Shutdown" ("State")] -> w104
      tunnel: [w338 w341 w388 w409 w431 w452 w474] -> w94
      tunnel: w98 -> [_ _ _ _ _ _ _]
      frame "Startup" {
        w338 = T38[] [enum."Reset Time"] items=["No Action", "Reset Time", "Reset All", "Open HW References", "Control FX Stop", "Control FX Mode 1", "Control FX Mode 2", "Set Robot Start Position", "Config HW Steer Set", "Config HW Steer Get", "Config HW Steer Save", "Config HW Steer Read", "Config HW Drive Set", "Config HW Drive Get", "Config HW Drive Save", "Config HW Drive Read", "Config HW Specific Set", "Config HW Specific Get", "Config HW Specific Save", "Config HW Specific Read", "Config System Save", "Config System Read", "Config From FP", "Start HW Steer Set", "Default HW Steer Set", "Defalut HW Drive Set"] ("Actions")
        n45 = call "Config Default.vi"() -> ("System Config Out"=w330:T15, "Drive Default Out"=w331:T1, "Steer Default Out"=w332:T6, "Module Specific Default Out"=w333:T12)  [unwired: 8 in]
        n46 = call "File RIO_Get or Create Team Folder.vi"() -> ("Team Files Folder"=w334:path)  [unwired: 10 in, 1 out]
        n47 = Bundle By Name(cluster=w335, "Team Folder"=w334, "Config Specific"=w333, "Config Steer"=w332, "Config Drive"=w331, "Config System"=w330) -> (w336:T37)
      }
      frame "Configuring" {
        w344 = T38[] [enum."Open HW References"] items=["No Action", "Reset Time", "Reset All", "Open HW References", "Control FX Stop", "Control FX Mode 1", "Control FX Mode 2", "Set Robot Start Position", "Config HW Steer Set", "Config HW Steer Get", "Config HW Steer Save", "Config HW Steer Read", "Config HW Drive Set", "Config HW Drive Get", "Config HW Drive Save", "Config HW Drive Read", "Config HW Specific Set", "Config HW Specific Get", "Config HW Specific Save", "Config HW Specific Read", "Config System Save", "Config System Read", "Config From FP", "Start HW Steer Set", "Default HW Steer Set", "Defalut HW Drive Set"] ("Action")
        w343 = T38[] [] items=["No Action", "Reset Time", "Reset All", "Open HW References", "Control FX Stop", "Control FX Mode 1", "Control FX Mode 2", "Set Robot Start Position", "Config HW Steer Set", "Config HW Steer Get", "Config HW Steer Save", "Config HW Steer Read", "Config HW Drive Set", "Config HW Drive Get", "Config HW Drive Save", "Config HW Drive Read", "Config HW Specific Set", "Config HW Specific Get", "Config HW Specific Save", "Config HW Specific Read", "Config System Save", "Config System Read", "Config From FP", "Start HW Steer Set", "Default HW Steer Set", "Defalut HW Drive Set"] ("Action")
        n48 = Unbundle By Name(w349) -> ("HW OPEN"=w345:bool, "Team Folder"=w340:path)
        n49 = Unbundle By Name(w349) -> ("Config Steer"=w361:T6)
        n50 = Unbundle By Name(w349) -> ("Config Specific"=w353:T12)
        n51 = Unbundle By Name(w349) -> ("Config Drive"=w356:T1)
        n52 = Unbundle By Name(w349) -> ("Config System"=w358:T15)
        n53 = call "Config_Build Name.vim"("Config First Name"=w356) -> ("Cfg file"=w355:string)  [unwired: 9 in, 1 out]
        n54 = call "Config_Build Name.vim"("Config First Name"=w361) -> ("Cfg file"=w363:string)  [unwired: 9 in, 1 out]
        n55 = call "Config_Build Name.vim"("Config First Name"=w358) -> ("Cfg file"=w359:string)  [unwired: 9 in, 1 out]
        n56 = call "Config_Build Name.vim"("Config First Name"=w353) -> ("Cfg file"=w351:string)  [unwired: 9 in, 1 out]
        n57 = Build Path(base path=w340, name or relative path=w359) -> (appended path=w357:path)
        n58 = Build Path(base path=w340, name or relative path=w355) -> (appended path=w354:path)
        n59 = Build Path(base path=w340, name or relative path=w351) -> (appended path=w352:path)
        n60 = Build Path(base path=w340, name or relative path=w363) -> (appended path=w362:path)
        n61 = call <vilib>:"Check if File or Folder Exists.vi"("path"=w357) -> ("file or folder exists?"=w348:bool)  [unwired: 8 in, 2 out]
        n62 = call <vilib>:"Check if File or Folder Exists.vi"("path"=w354) -> ("file or folder exists?"=w346:bool)  [unwired: 8 in, 2 out]
        n63 = call <vilib>:"Check if File or Folder Exists.vi"("path"=w352) -> ("file or folder exists?"=w350:bool)  [unwired: 8 in, 2 out]
        n64 = call <vilib>:"Check if File or Folder Exists.vi"("path"=w362) -> ("file or folder exists?"=w347:bool)  [unwired: 8 in, 2 out]
        n65 = Select(t=w343, s=w345, f=w344) -> (s? t:f=w342:T38[])
        n66 = Compound Arithmetic op=AND(w350, w348, w347, w346) -> (w339:bool)
        n67 = case shown="False" w339 {
          tunnel: [ENUM_ACT_State."Configuring" ("State") ENUM_ACT_State."Stopping" ("State")] -> w360
          tunnel: [w369 w386] -> w341
          tunnel: w350 -> [w382 _]
          tunnel: w348 -> [w378 _]
          tunnel: w347 -> [w376 _]
          tunnel: w346 -> [w371 _]
          tunnel: w342 -> [w364 w385]
          frame False {
            w373 = T38[] [enum."Config HW Drive Get", enum."Config HW Drive Save"] items=["No Action", "Reset Time", "Reset All", "Open HW References", "Control FX Stop", "Control FX Mode 1", "Control FX Mode 2", "Set Robot Start Position", "Config HW Steer Set", "Config HW Steer Get", "Config HW Steer Save", "Config HW Steer Read", "Config HW Drive Set", "Config HW Drive Get", "Config HW Drive Save", "Config HW Drive Read", "Config HW Specific Set", "Config HW Specific Get", "Config HW Specific Save", "Config HW Specific Read", "Config System Save", "Config System Read", "Config From FP", "Start HW Steer Set", "Default HW Steer Set", "Defalut HW Drive Set"] ("Action")
            w372 = T38[] [] items=["No Action", "Reset Time", "Reset All", "Open HW References", "Control FX Stop", "Control FX Mode 1", "Control FX Mode 2", "Set Robot Start Position", "Config HW Steer Set", "Config HW Steer Get", "Config HW Steer Save", "Config HW Steer Read", "Config HW Drive Set", "Config HW Drive Get", "Config HW Drive Save", "Config HW Drive Read", "Config HW Specific Set", "Config HW Specific Get", "Config HW Specific Save", "Config HW Specific Read", "Config System Save", "Config System Read", "Config From FP", "Start HW Steer Set", "Default HW Steer Set", "Defalut HW Drive Set"] ("Action")
            w374 = T38[] [enum."Config HW Steer Get", enum."Config HW Steer Save"] items=["No Action", "Reset Time", "Reset All", "Open HW References", "Control FX Stop", "Control FX Mode 1", "Control FX Mode 2", "Set Robot Start Position", "Config HW Steer Set", "Config HW Steer Get", "Config HW Steer Save", "Config HW Steer Read", "Config HW Drive Set", "Config HW Drive Get", "Config HW Drive Save", "Config HW Drive Read", "Config HW Specific Set", "Config HW Specific Get", "Config HW Specific Save", "Config HW Specific Read", "Config System Save", "Config System Read", "Config From FP", "Start HW Steer Set", "Default HW Steer Set", "Defalut HW Drive Set"] ("Action")
            w375 = T38[] [] items=["No Action", "Reset Time", "Reset All", "Open HW References", "Control FX Stop", "Control FX Mode 1", "Control FX Mode 2", "Set Robot Start Position", "Config HW Steer Set", "Config HW Steer Get", "Config HW Steer Save", "Config HW Steer Read", "Config HW Drive Set", "Config HW Drive Get", "Config HW Drive Save", "Config HW Drive Read", "Config HW Specific Set", "Config HW Specific Get", "Config HW Specific Save", "Config HW Specific Read", "Config System Save", "Config System Read", "Config From FP", "Start HW Steer Set", "Default HW Steer Set", "Defalut HW Drive Set"] ("Action")
            # "Config Files Missing"
            n68 = Select(t=w375, s=w376, f=w374) -> (s? t:f=w365:T38[])
            n69 = Select(t=ENUM_ACT_Action."No Action" ("Action"), s=w378, f=ENUM_ACT_Action."Config System Save" ("Action")) -> (s? t:f=w367:T38)
            n70 = Select(t=ENUM_ACT_Action."No Action" ("Action"), s=w382, f=ENUM_ACT_Action."Config HW Specific Save" ("Action")) -> (s? t:f=w366:T38)
            n71 = Select(t=w372, s=w371, f=w373) -> (s? t:f=w368:T38[])
            n72 = Build Array (concatenate)(w366, w367, w364, w365, w368) -> (w369:T38[])
          }
          frame True {
            w384 = T38[] [enum."Config HW Specific Read", enum."Config System Read", enum."Config HW Drive Read", enum."Config HW Steer Read"] items=["No Action", "Reset Time", "Reset All", "Open HW References", "Control FX Stop", "Control FX Mode 1", "Control FX Mode 2", "Set Robot Start Position", "Config HW Steer Set", "Config HW Steer Get", "Config HW Steer Save", "Config HW Steer Read", "Config HW Drive Set", "Config HW Drive Get", "Config HW Drive Save", "Config HW Drive Read", "Config HW Specific Set", "Config HW Specific Get", "Config HW Specific Save", "Config HW Specific Read", "Config System Save", "Config System Read", "Config From FP", "Start HW Steer Set", "Default HW Steer Set", "Defalut HW Drive Set"] ("Actions")
            w383 = T38[] [enum."Default HW Steer Set", enum."Defalut HW Drive Set", enum."Config HW Steer Set", enum."Config HW Specific Set", enum."Config HW Drive Set", enum."Start HW Steer Set"] items=["No Action", "Reset Time", "Reset All", "Open HW References", "Control FX Stop", "Control FX Mode 1", "Control FX Mode 2", "Set Robot Start Position", "Config HW Steer Set", "Config HW Steer Get", "Config HW Steer Save", "Config HW Steer Read", "Config HW Drive Set", "Config HW Drive Get", "Config HW Drive Save", "Config HW Drive Read", "Config HW Specific Set", "Config HW Specific Get", "Config HW Specific Save", "Config HW Specific Read", "Config System Save", "Config System Read", "Config From FP", "Start HW Steer Set", "Default HW Steer Set", "Defalut HW Drive Set"] ("Actions")
            # "All Config File are present"
            n73 = Build Array (concatenate)(w384, w385, w383) -> (w386:T38[])
          }
        }
      }
      frame "Stopping" {
        (unwired) TRUE
        w389 = T38[] [enum."Control FX Stop"] items=["No Action", "Reset Time", "Reset All", "Open HW References", "Control FX Stop", "Control FX Mode 1", "Control FX Mode 2", "Set Robot Start Position", "Config HW Steer Set", "Config HW Steer Get", "Config HW Steer Save", "Config HW Steer Read", "Config HW Drive Set", "Config HW Drive Get", "Config HW Drive Save", "Config HW Drive Read", "Config HW Specific Set", "Config HW Specific Get", "Config HW Specific Save", "Config HW Specific Read", "Config System Save", "Config System Read", "Config From FP", "Start HW Steer Set", "Default HW Steer Set", "Defalut HW Drive Set"] ("Actions")
        n74 = Unbundle By Name(w392) -> ("ACT Input.Mode"=w393:T27)
        n75 = case shown="\"STOP\"" w393 {
          tunnel: w392 -> [w396 w399 w402 w405 w408]
          tunnel: [w396 w399 w402 w405 w408] -> w391
          tunnel: [ENUM_ACT_State."Stopping" ("State") ENUM_ACT_State."Moving Mode 1" ("State") ENUM_ACT_State."Moving Mode 2" ("State") ENUM_ACT_State."Moving Mode 2" ("State") ENUM_ACT_State."Moving Mode 2" ("State")] -> w390
          tunnel: [w394 w397 w400 w403 w406] -> w388
          tunnel: w389 -> [w394 w397 w400 w403 w406]
          frame "STOP" {
          }
          frame "Move" {
          }
          frame "Turret Manual" {
          }
          frame "Trans Manual Angle Auto" {
          }
          frame "Turret Auto Angle" {
          }
        }
      }
      frame "Initializing HW" {
        (unwired) TRUE
        w410 = T38[] [enum."Control FX Stop"] items=["No Action", "Reset Time", "Reset All", "Open HW References", "Control FX Stop", "Control FX Mode 1", "Control FX Mode 2", "Set Robot Start Position", "Config HW Steer Set", "Config HW Steer Get", "Config HW Steer Save", "Config HW Steer Read", "Config HW Drive Set", "Config HW Drive Get", "Config HW Drive Save", "Config HW Drive Read", "Config HW Specific Set", "Config HW Specific Get", "Config HW Specific Save", "Config HW Specific Read", "Config System Save", "Config System Read", "Config From FP", "Start HW Steer Set", "Default HW Steer Set", "Defalut HW Drive Set"] ("Actions")
        n76 = Unbundle By Name(w413) -> ("ACT Input.Mode"=w414:T27)
        n77 = case shown="\"Trans Manual Angle Auto\"" w414 {
          tunnel: w413 -> [w417 w420 w423 w426 w429]
          tunnel: [w417 w420 w423 w426 w429] -> w412
          tunnel: [ENUM_ACT_State."Stopping" ("State") ENUM_ACT_State."Moving Mode 1" ("State") ENUM_ACT_State."Moving Mode 2" ("State") ENUM_ACT_State."Moving Mode 2" ("State") ENUM_ACT_State."Moving Mode 2" ("State")] -> w411
          tunnel: [w415 w418 w421 w424 w427] -> w409
          tunnel: w410 -> [w415 w418 w421 w424 w427]
          frame "STOP" {
          }
          frame "Move" {
          }
          frame "Turret Manual" {
          }
          frame "Trans Manual Angle Auto" {
          }
          frame "Turret Auto Angle" {
          }
        }
      }
      frame "Moving Mode 1" {
        w430 = T38[] [enum."Control FX Stop"] items=["No Action", "Reset Time", "Reset All", "Open HW References", "Control FX Stop", "Control FX Mode 1", "Control FX Mode 2", "Set Robot Start Position", "Config HW Steer Set", "Config HW Steer Get", "Config HW Steer Save", "Config HW Steer Read", "Config HW Drive Set", "Config HW Drive Get", "Config HW Drive Save", "Config HW Drive Read", "Config HW Specific Set", "Config HW Specific Get", "Config HW Specific Save", "Config HW Specific Read", "Config System Save", "Config System Read", "Config From FP", "Start HW Steer Set", "Default HW Steer Set", "Defalut HW Drive Set"] ("Actions")
        n78 = Unbundle By Name(w433) -> ("ACT Input.Mode"=w435:T27)
        n79 = case shown="\"Turret Auto Angle\"" w435 {
          tunnel: [ENUM_ACT_State."Stopping" ("State") ENUM_ACT_State."Moving Mode 2" ("State") ENUM_ACT_State."Moving Mode 2" ("State") ENUM_ACT_State."Moving Mode 2" ("State") w450] -> w436
          tunnel: w433 -> [w439 w442 w445 w448 w451]
          tunnel: [w439 w442 w445 w448 w451] -> w434
          tunnel: w432 -> [_ _ _ _ w450]
          tunnel: [w437 w440 w443 w446 w449] -> w431
          tunnel: w430 -> [w437 w440 w443 w446 _]
          frame "STOP" {
          }
          frame "Turret Manual" {
          }
          frame "Trans Manual Angle Auto" {
          }
          frame "Turret Auto Angle" {
          }
          frame "Move" {
            w449 = T38[] [enum."Control FX Mode 1"] items=["No Action", "Reset Time", "Reset All", "Open HW References", "Control FX Stop", "Control FX Mode 1", "Control FX Mode 2", "Set Robot Start Position", "Config HW Steer Set", "Config HW Steer Get", "Config HW Steer Save", "Config HW Steer Read", "Config HW Drive Set", "Config HW Drive Get", "Config HW Drive Save", "Config HW Drive Read", "Config HW Specific Set", "Config HW Specific Get", "Config HW Specific Save", "Config HW Specific Read", "Config System Save", "Config System Read", "Config From FP", "Start HW Steer Set", "Default HW Steer Set", "Defalut HW Drive Set"] ("Actions")
          }
        }
      }
      frame "Moving Mode 2" {
        w453 = T38[] [enum."Control FX Stop"] items=["No Action", "Reset Time", "Reset All", "Open HW References", "Control FX Stop", "Control FX Mode 1", "Control FX Mode 2", "Set Robot Start Position", "Config HW Steer Set", "Config HW Steer Get", "Config HW Steer Save", "Config HW Steer Read", "Config HW Drive Set", "Config HW Drive Get", "Config HW Drive Save", "Config HW Drive Read", "Config HW Specific Set", "Config HW Specific Get", "Config HW Specific Save", "Config HW Specific Read", "Config System Save", "Config System Read", "Config From FP", "Start HW Steer Set", "Default HW Steer Set", "Defalut HW Drive Set"] ("Actions")
        n80 = Unbundle By Name(w455) -> ("ACT Input.Mode"=w457:T27)
        n81 = case shown="\"Turret Auto Angle\"" w457 {
          tunnel: [ENUM_ACT_State."Stopping" ("State") w462 w465 w468 ENUM_ACT_State."Moving Mode 1" ("State")] -> w458
          tunnel: w455 -> [w461 w464 w467 w470 w473]
          tunnel: [w461 w464 w467 w470 w473] -> w456
          tunnel: w454 -> [_ w462 w465 w468 _]
          tunnel: [w459 w463 w466 w469 w471] -> w452
          tunnel: w453 -> [w459 _ _ _ w471]
          frame "STOP" {
          }
          frame "Turret Manual" {
            w463 = T38[] [enum."Control FX Mode 2"] items=["No Action", "Reset Time", "Reset All", "Open HW References", "Control FX Stop", "Control FX Mode 1", "Control FX Mode 2", "Set Robot Start Position", "Config HW Steer Set", "Config HW Steer Get", "Config HW Steer Save", "Config HW Steer Read", "Config HW Drive Set", "Config HW Drive Get", "Config HW Drive Save", "Config HW Drive Read", "Config HW Specific Set", "Config HW Specific Get", "Config HW Specific Save", "Config HW Specific Read", "Config System Save", "Config System Read", "Config From FP", "Start HW Steer Set", "Default HW Steer Set", "Defalut HW Drive Set"] ("Actions")
          }
          frame "Trans Manual Angle Auto" {
            w466 = T38[] [enum."Control FX Mode 2"] items=["No Action", "Reset Time", "Reset All", "Open HW References", "Control FX Stop", "Control FX Mode 1", "Control FX Mode 2", "Set Robot Start Position", "Config HW Steer Set", "Config HW Steer Get", "Config HW Steer Save", "Config HW Steer Read", "Config HW Drive Set", "Config HW Drive Get", "Config HW Drive Save", "Config HW Drive Read", "Config HW Specific Set", "Config HW Specific Get", "Config HW Specific Save", "Config HW Specific Read", "Config System Save", "Config System Read", "Config From FP", "Start HW Steer Set", "Default HW Steer Set", "Defalut HW Drive Set"] ("Actions")
          }
          frame "Turret Auto Angle" {
            w469 = T38[] [enum."Control FX Mode 2"] items=["No Action", "Reset Time", "Reset All", "Open HW References", "Control FX Stop", "Control FX Mode 1", "Control FX Mode 2", "Set Robot Start Position", "Config HW Steer Set", "Config HW Steer Get", "Config HW Steer Save", "Config HW Steer Read", "Config HW Drive Set", "Config HW Drive Get", "Config HW Drive Save", "Config HW Drive Read", "Config HW Specific Set", "Config HW Specific Get", "Config HW Specific Save", "Config HW Specific Read", "Config System Save", "Config System Read", "Config From FP", "Start HW Steer Set", "Default HW Steer Set", "Defalut HW Drive Set"] ("Actions")
          }
          frame "Move" {
          }
        }
      }
      frame "Shutdown" {
        w474 = T38[] [enum."Reset All"] items=["No Action", "Reset Time", "Reset All", "Open HW References", "Control FX Stop", "Control FX Mode 1", "Control FX Mode 2", "Set Robot Start Position", "Config HW Steer Set", "Config HW Steer Get", "Config HW Steer Save", "Config HW Steer Read", "Config HW Drive Set", "Config HW Drive Get", "Config HW Drive Save", "Config HW Drive Read", "Config HW Specific Set", "Config HW Specific Get", "Config HW Specific Save", "Config HW Specific Read", "Config System Save", "Config System Read", "Config From FP", "Start HW Steer Set", "Default HW Steer Set", "Defalut HW Drive Set"] ("Actions")
      }
    }
    n82 = case shown="True" w77 {
      tunnel: w76 -> [_ w479]
      tunnel: [_ w477] -> w75
      frame False {
      }
      frame True {
        n83 = call "Search Unsorted 1D Array.vim"("element"=TRUE, "unsorted 1D array"=w479) -> ("index of element"=w478:i32)  [unwired: 9 in]
        n84 = case shown="5" w478 {
          tunnel: [w481 w482 w483 w484 w485 w486 w487] -> w477
          frame ..0 {
            w481 = T38[] [enum."Config HW Specific Read", enum."Config HW Steer Read", enum."Config HW Drive Read", enum."Config System Read"] items=["No Action", "Reset Time", "Reset All", "Open HW References", "Control FX Stop", "Control FX Mode 1", "Control FX Mode 2", "Set Robot Start Position", "Config HW Steer Set", "Config HW Steer Get", "Config HW Steer Save", "Config HW Steer Read", "Config HW Drive Set", "Config HW Drive Get", "Config HW Drive Save", "Config HW Drive Read", "Config HW Specific Set", "Config HW Specific Get", "Config HW Specific Save", "Config HW Specific Read", "Config System Save", "Config System Read", "Config From FP", "Start HW Steer Set", "Default HW Steer Set", "Defalut HW Drive Set"] ("Actions")
            # "Read Config"
          }
          frame 1 {
            w482 = T38[] [enum."Config From FP"] items=["No Action", "Reset Time", "Reset All", "Open HW References", "Control FX Stop", "Control FX Mode 1", "Control FX Mode 2", "Set Robot Start Position", "Config HW Steer Set", "Config HW Steer Get", "Config HW Steer Save", "Config HW Steer Read", "Config HW Drive Set", "Config HW Drive Get", "Config HW Drive Save", "Config HW Drive Read", "Config HW Specific Set", "Config HW Specific Get", "Config HW Specific Save", "Config HW Specific Read", "Config System Save", "Config System Read", "Config From FP", "Start HW Steer Set", "Default HW Steer Set", "Defalut HW Drive Set"] ("Actions")
            # "Updated Config"
          }
          frame 2 {
            w483 = T38[] [enum."Config HW Steer Set", enum."Config HW Steer Save"] items=["No Action", "Reset Time", "Reset All", "Open HW References", "Control FX Stop", "Control FX Mode 1", "Control FX Mode 2", "Set Robot Start Position", "Config HW Steer Set", "Config HW Steer Get", "Config HW Steer Save", "Config HW Steer Read", "Config HW Drive Set", "Config HW Drive Get", "Config HW Drive Save", "Config HW Drive Read", "Config HW Specific Set", "Config HW Specific Get", "Config HW Specific Save", "Config HW Specific Read", "Config System Save", "Config System Read", "Config From FP", "Start HW Steer Set", "Default HW Steer Set", "Defalut HW Drive Set"] ("Actions")
            # "Steer Change"
          }
          frame 3 {
            w484 = T38[] [enum."Config HW Drive Set", enum."Config HW Drive Save"] items=["No Action", "Reset Time", "Reset All", "Open HW References", "Control FX Stop", "Control FX Mode 1", "Control FX Mode 2", "Set Robot Start Position", "Config HW Steer Set", "Config HW Steer Get", "Config HW Steer Save", "Config HW Steer Read", "Config HW Drive Set", "Config HW Drive Get", "Config HW Drive Save", "Config HW Drive Read", "Config HW Specific Set", "Config HW Specific Get", "Config HW Specific Save", "Config HW Specific Read", "Config System Save", "Config System Read", "Config From FP", "Start HW Steer Set", "Default HW Steer Set", "Defalut HW Drive Set"] ("Actions")
            # "Drive Change"
          }
          frame 4 {
            w485 = T38[] [enum."Config HW Specific Save"] items=["No Action", "Reset Time", "Reset All", "Open HW References", "Control FX Stop", "Control FX Mode 1", "Control FX Mode 2", "Set Robot Start Position", "Config HW Steer Set", "Config HW Steer Get", "Config HW Steer Save", "Config HW Steer Read", "Config HW Drive Set", "Config HW Drive Get", "Config HW Drive Save", "Config HW Drive Read", "Config HW Specific Set", "Config HW Specific Get", "Config HW Specific Save", "Config HW Specific Read", "Config System Save", "Config System Read", "Config From FP", "Start HW Steer Set", "Default HW Steer Set", "Defalut HW Drive Set"] ("Actions")
            # "Specific Change"
          }
          frame 5 {
            w486 = T38[] [enum."Config System Save"] items=["No Action", "Reset Time", "Reset All", "Open HW References", "Control FX Stop", "Control FX Mode 1", "Control FX Mode 2", "Set Robot Start Position", "Config HW Steer Set", "Config HW Steer Get", "Config HW Steer Save", "Config HW Steer Read", "Config HW Drive Set", "Config HW Drive Get", "Config HW Drive Save", "Config HW Drive Read", "Config HW Specific Set", "Config HW Specific Get", "Config HW Specific Save", "Config HW Specific Read", "Config System Save", "Config System Read", "Config From FP", "Start HW Steer Set", "Default HW Steer Set", "Defalut HW Drive Set"] ("Actions")
            # "System Change"
          }
          frame 6.. {
            w487 = T38[] [enum."Config HW Specific Get"] items=["No Action", "Reset Time", "Reset All", "Open HW References", "Control FX Stop", "Control FX Mode 1", "Control FX Mode 2", "Set Robot Start Position", "Config HW Steer Set", "Config HW Steer Get", "Config HW Steer Save", "Config HW Steer Read", "Config HW Drive Set", "Config HW Drive Get", "Config HW Drive Save", "Config HW Drive Read", "Config HW Specific Set", "Config HW Specific Get", "Config HW Specific Save", "Config HW Specific Read", "Config System Save", "Config System Read", "Config From FP", "Start HW Steer Set", "Default HW Steer Set", "Defalut HW Drive Set"] ("Actions")
            # "System Change"
          }
        }
      }
    }
    n85 = global write "Global_ACT_Data Out.vi" "ACT_Template_STATE"(w65) -> ()
    n86 = Bundle By Name(cluster=w105, "Previous State"=w65, "State"=w104) -> (w106:T37)
    n87 = Build Array (concatenate)(w94, w75) -> (w90:T38[])
    n88 = for {
      tunnel: w90 -> [w138] mode=indexing
      shift-right: [w137] -> w89
      shift-left: w106 -> [w136]
      n89 = case shown="\"Defalut HW Drive Set\"" w138 {
        tunnel: w136 -> [w139 w142 w143 w148 w155 w156 w157 w158 w160 w174 w188 w196 w199 w212 w226 w234 w240 w251 w263 w270 w277 w284 w297 w315 w317 w324]
        tunnel: [w139 w141 w143 w149 w155 w156 w157 w158 w159 w173 w189 w197 w198 w211 w227 w235 w242 w253 w264 w271 w278 w285 w298 w315 w316 w323] -> w137
        frame "No Action" {
        }
        frame "Reset Time" {
          n90 = Unbundle By Name(w142) -> ("Current Time"=w140:timestamp)
          n91 = Bundle By Name(cluster=w142, "Start Time"=w140) -> (w141:T37)
        }
        frame "Reset All" {
        }
        frame "Open HW References" {
          n92 = Unbundle By Name(w148) -> ("Config Specific.Specific Data"=w147:T13[])
          n93 = for {
            tunnel: w147 -> [w154] mode=indexing
            tunnel: [w152] -> w146 mode=indexing
            tunnel: [w153] -> w145 mode=indexing
            tunnel: [w151] -> _
            tunnel: [w150] -> _
            n94 = call "Open HW References.vi"("Module Azimuth Config Data"=w154) -> (0:"Error Out"=w151:errorcluster, 1:"Error Out"=w150:errorcluster, "Module Drive Ref Out"=w153:T30, "Module Steer Ref Out"=w152:T30)  [unwired: 7 in]
          }
          n95 = Bundle By Name(cluster=w148, "Steer Refs"=w146, "Drive Refs"=w145, "HW OPEN"=TRUE) -> (w149:T37)
        }
        frame "Control FX Stop" {
          # "#Fix"
        }
        frame "Control FX Mode 1" {
          # "#Fix"
        }
        frame "Control FX Mode 2" {
          # "#Fix"
        }
        frame "Set Robot Start Position" {
          # "#Fix"
        }
        frame "Config HW Steer Set" {
          n96 = in-place {
            n97 = in-place-cluster #1(w160) -> ("Config Steer"=w163:T6, "Steer Refs"=w165:T30[])  [unwired: 1 out]
            n98 = for {
              tunnel: w165 -> [w172] mode=indexing
              tunnel: [w171] -> w164 mode=indexing
              shift-right: [w169] -> w162
              shift-left: w163 -> [w170]
              n99 = call "Config Steer Module Get-Set.vi"("Start With Default"=FALSE, "Get(f) Set(t)"=TRUE, "Set Steer Values"=w170, "Send Cmd Timout(ms)"=u32 300, "Steer Refs"=w172) -> ("Steer Refs Out"=w171:T30, "Steer Config Out"=w169:T6)  [unwired: 3 in, 2 out]
            }
            n100 = in-place-cluster #1("Config Steer"=w162, "Steer Refs"=w164, "Steer Change"=FALSE ("Update Display")) -> (w159:T37)
          }
        }
        frame "Config HW Steer Get" {
          n101 = in-place {
            n102 = in-place-cluster #2(w174) -> ("Config Steer"=w182:T6, "Steer Refs"=w176:T30[])  [unwired: 1 out]
            n103 = Index Array(array=w176) -> (element=w177:T30)  [unwired: 1 in]
            n104 = call "Config Steer Module Get-Set.vi"("Start With Default"=FALSE, "Get(f) Set(t)"=FALSE, "Set Steer Values"=w182, "Send Cmd Timout(ms)"=u32 300, "Steer Refs"=w177) -> ("Steer Config Out"=w181:T6)  [unwired: 3 in, 3 out]
            n105 = in-place-cluster #2("Config Steer"=w181, "Steer Refs"=w176, "Update Display"=TRUE) -> (w173:T37)
          }
        }
        frame "Config HW Steer Save" {
          n106 = Unbundle By Name(w188) -> ("Team Folder"=w185:path, "Config Steer"=w187:T6)
          n107 = call "RWA_File Config.vim"("Read(f) Save(t)"=TRUE ("Read(f) Write(t)"), "Target Folder Folder"=w185, "Any Config"=w187) -> ("Any Config Out"=w186:T6)  [unwired: 4 in, 4 out]
          n108 = Bundle By Name(cluster=w188, "Config Steer"=w186, "Steer Change"=FALSE) -> (w189:T37)
        }
        frame "Config HW Steer Read" {
          n109 = Unbundle By Name(w196) -> ("Team Folder"=w195:path, "Config Steer"=w191:T6)
          n110 = call "RWA_File Config.vim"("Read(f) Save(t)"=FALSE ("Read(f) Write(t)"), "Target Folder Folder"=w195, "Any Config"=w191) -> ("Any Config Out"=w192:T6)  [unwired: 4 in, 4 out]
          n111 = Not Equal?(x=w191, y=w192) -> (x != y?=w190:bool)
          n112 = Bundle By Name(cluster=w196, "Steer Change"=w190, "Config Steer"=w192, "Update Display"=TRUE) -> (w197:T37)
        }
        frame "Config HW Drive Set" {
          n113 = in-place {
            n114 = in-place-cluster #3(w199) -> ("Config Drive"=w202:T1, "Drive Refs"=w204:T30[])  [unwired: 1 out]
            n115 = for {
              tunnel: w204 -> [w210] mode=indexing
              tunnel: [w209] -> w203 mode=indexing
              shift-right: [w207] -> w201
              shift-left: w202 -> [w208]
              n116 = call "Config Drive Module Get-Set.vi"("Start with Default"=FALSE ("Start With Default"), "Get(f) Set(t)"=TRUE, "Set Drive Config"=w208, "Drive Refs"=w210) -> ("Drive Refs Out"=w209:T30, "Drive Config Out"=w207:T1)  [unwired: 5 in, 1 out]
            }
            n117 = in-place-cluster #3("Config Drive"=w201, "Drive Refs"=w203, "Drive Change"=FALSE) -> (w198:T37)
          }
        }
        frame "Config HW Drive Get" {
          n118 = in-place {
            n119 = in-place-cluster #4(w212) -> ("Config Drive"=w220:T1, "Drive Refs"=w215:T30[])  [unwired: 1 out]
            n120 = Index Array(array=w215, index=3) -> (element=w216:T30)
            n121 = call "Config Drive Module Get-Set.vi"("Start with Default"=FALSE ("Start With Default"), "Get(f) Set(t)"=FALSE, "Set Drive Config"=w220, "Drive Refs"=w216) -> ("Drive Config Out"=w219:T1)  [unwired: 5 in, 2 out]
            n122 = in-place-cluster #4("Config Drive"=w219, "Drive Refs"=w215, "Update Display"=TRUE) -> (w211:T37)
          }
        }
        frame "Config HW Drive Save" {
          n123 = Unbundle By Name(w226) -> ("Team Folder"=w223:path, "Config Drive"=w225:T1)
          n124 = call "RWA_File Config.vim"("Read(f) Save(t)"=TRUE ("Read(f) Write(t)"), "Target Folder Folder"=w223, "Any Config"=w225) -> ("Any Config Out"=w224:T1)  [unwired: 4 in, 4 out]
          n125 = Bundle By Name(cluster=w226, "Config Drive"=w224, "Drive Change"=FALSE) -> (w227:T37)
        }
        frame "Config HW Drive Read" {
          n126 = Unbundle By Name(w234) -> ("Team Folder"=w233:path, "Config Drive"=w229:T1)
          n127 = call "RWA_File Config.vim"("Read(f) Save(t)"=FALSE ("Read(f) Write(t)"), "Target Folder Folder"=w233, "Any Config"=w229) -> ("Any Config Out"=w230:T1)  [unwired: 4 in, 4 out]
          n128 = Not Equal?(x=w229, y=w230) -> (x != y?=w228:bool)
          n129 = Bundle By Name(cluster=w234, "Drive Change"=w228, "Config Drive"=w230, "Update Display"=TRUE) -> (w235:T37)
        }
        frame "Config HW Specific Set" {
          n130 = Unbundle By Name(w240) -> ("Config Specific.Specific Data"=w238:T13[], "HW Out.Swerve Read"=w239:T23)
          n131 = Cluster To Array(cluster=w239) -> (array=w236:T24[])
          n132 = for {
            tunnel: w238 -> [w245] mode=indexing
            tunnel: [w246] -> w237 mode=indexing
            tunnel: w236 -> [w244] mode=indexing
            n133 = Unbundle By Name(w244) -> ("Angle"=w243:T22)
            n134 = Bundle By Name(cluster=w245, "Encoder Start Value"=w243) -> (w246:T13)
          }
          n135 = Bundle By Name(cluster=w240, "Config Specific.Specific Data"=w237, "Specific Change"=TRUE) -> (w242:T37)
        }
        frame "Config HW Specific Get" {
          n136 = Unbundle By Name(w251) -> ("Config Specific.Specific Data"=w249:T13[], "HW Out.Swerve Read"=w250:T23)
          n137 = Cluster To Array(cluster=w250) -> (array=w247:T24[])
          n138 = for {
            tunnel: w249 -> [w256] mode=indexing
            tunnel: [w257] -> w248 mode=indexing
            tunnel: w247 -> [w255] mode=indexing
            n139 = Unbundle By Name(w255) -> ("Angle"=w254:T22)
            n140 = Bundle By Name(cluster=w256, "Encoder Start Value"=w254) -> (w257:T13)
          }
          n141 = Bundle By Name(cluster=w251, "Config Specific.Specific Data"=w248, "Specific Change"=TRUE) -> (w253:T37)
        }
        frame "Config HW Specific Save" {
          n142 = Unbundle By Name(w263) -> ("Team Folder"=w260:path, "Config Specific"=w262:T12)
          n143 = call "RWA_File Config.vim"("Read(f) Save(t)"=TRUE ("Read(f) Write(t)"), "Target Folder Folder"=w260, "Any Config"=w262) -> ("Any Config Out"=w261:T12)  [unwired: 4 in, 4 out]
          n144 = Bundle By Name(cluster=w263, "Config Specific"=w261, "Specific Change"=FALSE) -> (w264:T37)
        }
        frame "Config HW Specific Read" {
          n145 = Unbundle By Name(w270) -> ("Team Folder"=w267:path, "Config System"=w269:T15)
          n146 = call "RWA_File Config.vim"("Read(f) Save(t)"=FALSE ("Read(f) Write(t)"), "Target Folder Folder"=w267, "Any Config"=w269) -> ("Any Config Out"=w268:T15)  [unwired: 4 in, 4 out]
          n147 = Bundle By Name(cluster=w270, "Config System"=w268, "Update Display"=TRUE) -> (w271:T37)
        }
        frame "Config System Save" {
          n148 = Unbundle By Name(w277) -> ("Team Folder"=w274:path, "Config System"=w276:T15)
          n149 = call "RWA_File Config.vim"("Read(f) Save(t)"=TRUE ("Read(f) Write(t)"), "Target Folder Folder"=w274, "Any Config"=w276) -> ("Any Config Out"=w275:T15)  [unwired: 4 in, 4 out]
          n150 = Bundle By Name(cluster=w277, "Config System"=w275, "System Change"=FALSE) -> (w278:T37)
        }
        frame "Config System Read" {
          n151 = Unbundle By Name(w284) -> ("Team Folder"=w281:path, "Config System"=w283:T15)
          n152 = call "RWA_File Config.vim"("Read(f) Save(t)"=FALSE ("Read(f) Write(t)"), "Target Folder Folder"=w281, "Any Config"=w283) -> ("Any Config Out"=w282:T15)  [unwired: 4 in, 4 out]
          n153 = Bundle By Name(cluster=w284, "Config System"=w282, "Update Display"=TRUE) -> (w285:T37)
        }
        frame "Config From FP" {
          n154 = Unbundle By Name(w297) -> ("Current Time"=w314:timestamp)
          n155 = Unbundle By Name(w297) -> ("Config Drive"=w303:T1, "Config Drive.Drive HW Ver"=w301:u64, "Config Steer"=w302:T6, "Config Steer.Steer HW Ver"=w299:u64)
          n156 = Unbundle By Name(w297) -> ("Config Specific"=w308:T12, "Config Specific.Specific HW Ver"=w307:u64)
          n157 = Unbundle By Name(w297) -> ("Config System"=w309:T15, "Config System.System Ver"=w311:u64)
          n158 = call "Date Stamp.vi"("Time"=w314) -> ("U64 Out"=w300:u64)  [unwired: 5 in, 1 out]
          n159 = Not Equal?(x=w309, y="Config System") -> (x != y?=w289:bool)
          n160 = Not Equal?(x="Config Specific", y=w308) -> (x != y?=w286:bool)
          n161 = Select(t=w300, s=w289, f=w311) -> (s? t:f=w310:u64)
          n162 = Select(t=w300, s=w286, f=w307) -> (s? t:f=w305:u64)
          n163 = Not Equal?(x="Config Steer", y=w302) -> (x != y?=w287:bool)
          n164 = Bundle By Name(cluster="Config System", "System Ver"=w310) -> (w313:T15)
          n165 = Not Equal?(x="Config Drive", y=w303) -> (x != y?=w290:bool)
          n166 = Select(t=w300, s=w287, f=w299) -> (s? t:f=w291:u64)
          n167 = Bundle By Name(cluster="Config Steer", "Steer HW Ver"=w291) -> (w292:T6)
          n168 = Bundle By Name(cluster="Config Specific", "Specific HW Ver"=w305) -> (w304:T12)
          n169 = Select(t=w300, s=w290, f=w301) -> (s? t:f=w295:u64)
          n170 = Bundle By Name(cluster="Config Drive", "Drive HW Ver"=w295) -> (w294:T1)
          n171 = Bundle By Name(cluster=w297, "Config Drive"=w294, "Drive Change"=w290, "Config Steer"=w292, "Steer Change"=w287, "Config System"=w313, "System Change"=w289, "Config Specific"=w304, "Specific Change"=w286, "Update Display"=TRUE) -> (w298:T37)
        }
        frame "Start HW Steer Set" {
        }
        frame "Default HW Steer Set" {
          n172 = in-place {
            w318 = TRUE ("Drive Change")
            n173 = in-place-cluster #5(w317) -> ("Steer Refs"=w320:T30[])  [unwired: 2 out]
            n174 = for {
              tunnel: w320 -> [w322] mode=indexing
              tunnel: [w321] -> w319 mode=indexing
              n175 = call <vilib>:"CTRE_Phoenix_MotorControl_FactoryDefault.vi"("PhoenixMotorControlDevRef"=w322) -> ("PhoenixMotorControlDevRef"=w321:T30)  [unwired: 9 in, 1 out]
            }
            n176 = in-place-cluster #5("Steer Refs"=w319, "Steer Change"=w318, "Specific Change"=w318) -> (w316:T37)
          }
        }
        frame "Defalut HW Drive Set" {
          n177 = in-place {
            n178 = in-place-cluster #6(w324) -> ("Drive Refs"=w327:T30[])  [unwired: 1 out]
            n179 = for {
              tunnel: w327 -> [w329] mode=indexing
              tunnel: [w328] -> w326 mode=indexing
              n180 = call <vilib>:"SPARK Restore Factory Default.vi"("MotorControlDeviceRef"=w329) -> ("MotorControlDeviceRef"=w328:T30)  [unwired: 9 in, 1 out]
            }
            n181 = in-place-cluster #6("Drive Refs"=w326, "Drive Change"=TRUE) -> (w323:T37)
          }
        }
      }
    }
    n182 = Unbundle By Name(w89) -> ("Config System"=w45:T15, "Config Drive"=w46:T1, "Config Steer"=w86:T6, "Update Display"=w87:bool, "Config System"=w69:T15, "Config Specific"=w53:T12)
    n183 = Unbundle By Name(w89) -> ("State"=w85:T36)
    n184 = Unbundle By Name(w89) -> ("Cycle Time(S)"=w91:dbl)
    "Cycle Time (S)" <- w91
    n185 = Unbundle By Name(w89) -> ("ACT Input"=→"CMD":T26, "HW Out"=w83:T21, "System Output"=w74:T20)
    "HW Output" <- w83
    "System Config" <- w74
    n186 = case shown="\"Startup\", \"Configuring\"" w85 {
      frame "Startup", "Configuring" {
        # "#Fix"
      }
      frame Default {
      }
    }
    n187 = case shown="False" w87 {
      tunnel: w86 -> [_ w490]
      tunnel: w69 -> [_ w492]
      tunnel: w53 -> [_ w491]
      tunnel: w46 -> [_ w489]
      tunnel: w45 -> [_ w488]
      frame False {
      }
      frame True {
        n188 = local write "Config System"(w492) -> ()
        n189 = local write "Config Specific"(w491) -> ()
        n190 = local write "Config Steer"(w490) -> ()
        n191 = local write "Config System"(w488) -> ()
        n192 = local write "Config Drive"(w489) -> ()
      }
    }
    n193 = global write "Global_ACT_Data Out.vi" "ACT_Template_System Output"(w74) -> ()
    n194 = global write "Global_ACT_Data Out.vi" "ACT_Template_HW Output"(w83) -> ()
    n195 = global write "Global_ACT_Data Out.vi" "ACT_Template_CycleTime(S)"(w91) -> ()
    n196 = Bundle By Name(cluster=w89, "Update Display"=FALSE) -> (w92:T37)
  }
  n197 = flat-sequence {
    frame #0 {
      (unwired) ENUM_ACT_State."Startup" ("State")
      (unwired) ENUM_ACT_Action."No Action" ("Action")
      # "State LIST"
      # "Action LIST"
    }
  }
  n198 = Unbundle By Name(w28) -> ("Steer Refs"=w25:T30[], "Drive Refs"=w13:T30[])
  n199 = for {
    tunnel: w25 -> [w494] mode=indexing
    tunnel: w13 -> [w493] mode=indexing
    n200 = call <vilib>:"WPI_MotorControlDisable.vi"("MotorControlDevRef"=w493) -> ()  [unwired: 9 in, 2 out]
    n201 = call <vilib>:"WPI_MotorControlDisable.vi"("MotorControlDevRef"=w494) -> ()  [unwired: 9 in, 2 out]
  }
